vi "SPS Flow System Automation.vi"() -> ()   [LabVIEW 2018]
uses:
  Serial configuration cluster control.ctl
  SPS Flow System Automation Control.ctl
  <vilib>/Utility/miscctls.llb/LVRowAndColumnTypeDef.ctl
panel:
  out "Path to ConditionTable (*.txt)":path caption="selected path"
  in  "Left Syringe Type":u16(ring)=2500 items=["Yellow Syringes"=50, "Green Syringes"=250, "Blue Syringes"=500, "Red Syringes"=2500]
  in  "Right Syringe Type":u16(ring)=500 items=["Yellow Syringes"=50, "Green Syringes"=250, "Blue Syringes"=500, "Red Syringes"=2500]
  out "State":T1=enum."Check temp & time "
  in  "Simulate Right Pump":i32(ring)=2 items=["Error"=-1, "Unitialised"=0, "Initialising"=1, "Idle"=2, "Filling"=3, "Full"=4, "Emptying"=5, "Empty"=6, "Pumping"=7]
  out "Pump2-2":bool
  out "Status":i32(ring) items=["Error"=-1, "Unitialised"=0, "Initialising"=1, "Idle"=2, "Filling"=3, "Full"=4, "Emptying"=5, "Empty"=6, "Pumping"=7]
  out "Pump2-1":bool
  in  "Waste Port (Valve 4)":u32=1
  out "Flow Rate\n(ml/min)":sgl
  in  "Temp range":dbl=5.0 caption="Temp(°C) Range ±"
  out "Asia pump connection":i32
  in  "Simulate Left Pump":i32(ring)=2 items=["Error"=-1, "Unitialised"=0, "Initialising"=1, "Idle"=2, "Filling"=3, "Full"=4, "Emptying"=5, "Empty"=6, "Pumping"=7]
  out "Flow Rate\n(ml/min)":sgl
  out "Status":i32(ring) items=["Error"=-1, "Unitialised"=0, "Initialising"=1, "Idle"=2, "Filling"=3, "Full"=4, "Emptying"=5, "Empty"=6, "Pumping"=7]
  out "Valve 4":u32(knob) scale=10.0..1.0
  out "Current Temp":dbl(slide) scale=10.0..150.0
  out "Pump1":bool
  in  "Valve pos reached":bool
  in  "temp reached":bool
  in  "Starting from row":i32=1
  out "Conditions Table":string[][](table)=[["1-1 1st reaction", "0.5", "2", "2", "0", "0", "10", "1", "1", "off", "off"], ["1-2 heating", "x", "0", "2", "0", "0", "10", "1", "1", "32", "500"], ["1-2 1st reaction", "0.5", "4", "2", "0", "0", "10", "1", "1", "32", "500"], ["1-3 DCM wash", "0.5", "5", "1", "0", "0", "10", "2", "1", "off", "off"], ["1-4 MeOH wash", "0.5", "2", "7", "0", "0", "10", "2", "1", "off", "off"], ["1-5 N2 purge", "0.5", "0", "6", "0", "0", "10", "2", "10", "off", "off"], ["1-6 THF wash", "0.5", "1", "6", "1", "1", "10", "2", "1", "off", "off"], ["1-7 THF wash", "0.5", "2", "6", "3", "1", "10", "2", "1", "off", "off"], ["2-1 2nd mixing", "0.5", "2.5", "3", "2.5", "0", "9", "3", "1", "off", "off"], ["2-2 heating", "x", "0", "4", "0", "0", "9", "3", "1", "38", "500"], ["2-3 2nd reaction", "0.5", "3", "4", "0", "0", "9", "3", "1", "38", "500"], ["2-5 THF wash", "0.5", "2", "6", "1", "1", "10", "2", "1", "38", "500"], ["2-4 N2 purge", "0.5", "0", "6", "0", "0", "10", "2", "10", "38", "500"], ["2-6 cooling", "x", "0", "6", "0", "0", "10", "2", "1", "30", "500"], ["2-7 THF wash", "0.5", "2.5", "6", "2.5", "1", "10", "2", "1", "off", "off"], ["3-1 3rd reaction", "0.5", "2.5", "5", "0", "2.5", "1", "2", "1", "off", "off"], ["3-3 THF wash", "0.5", "2.5", "6", "1", "2.5", "10", "2", "1", "off", "off"], ["3-4 0.5 N HCl wash", "0.5", "0", "6", "5", "0", "7", "2", "1", "off", "off"], ["3-6 heating", "x", "0", "6", "0", "0", "7", "2", "1", "60", "500"], ["3-7 H2O wash", "20", "0", "6", "5", "0", "8", "2", "1", "60", "500"], ["3-8 THF wash", "15", "0", "6", "4", "1", "10", "2", "1", "60", "500"], ["4-1 EtOH-THF wash", "20", "0", "6", "2.5", "0", "3", "2", "1", "60", "500"], ["4-1 heating", "x", "0", "6", "0", "0", "3", "5", "1", "110", "500"], ["4-3 4th reaction", "360", "0", "6", "2.5", "0", "2", "4", "1", "110", "500"], ["4-4 EtOH-THF wash ", "20", "0", "6", "2.5", "0", "3", "5", "1", "110", "500"], ["4-5 THF wash  ", "20", "1.5", "6", "2.5", "1", "10", "5", "1", "110", "500"], ["4-6 N2 purge", "20", "0", "6", "0", "0", "10", "2", "10", "110", "500"], ["5-1 Dioxane-DMSO wash", "20", "2.5", "15", "2.5", "0", "4", "5", "1", "110", "500"], ["5-2 5th mixing", "12", "2.5", "14", "2.5", "0", "5", "6", "1", "110", "500"], ["5-3 5th reaction", "600", "0", "14", "2.5", "0", "6", "6", "1", "110", "500"], ["5-4 MeOH & THF wash", "20", "2.5", "7", "1.5", "1", "10", "5", "1", "off", "off"], ["5-5 N2 purge", "20", "0", "7", "0", "0", "10", "2", "10", "off", "off"], ["6-1 DCM wash", "15", "2", "1", "0", "0", "10", "2", "1", "off", "off"], ["6-2 DCM wash", "20", "5", "1", "0", "0", "10", "2", "1", "off", "off"], ["6-4 6th reaction", "60", "3", "16", "0", "0", "10", "7", "1", "off", "off"], ["6-5 DCM wash", "10", "5", "1", "0", "0", "10", "7", "1", "off", "off"], ["", "", "", "", "", "", "", "", "", "", ""], ["", "", "", "", "", "", "", "", "", "", ""], ["", "", "", "", "", "", "", "", "", "", ""], ["", "", "", "", "", "", "", "", "", "", ""], ["", "", "", "", "", "", "", "", "", "", ""], ["", "", "", "", "", "", "", "", "", "", ""], ["", "", "", "", "", "", "", "", "", "", ""], ["", "", "", "", "", "", "", "", "", "", ""], ["", "", "", "", "", "", "", "", "", "", ""], ["", "", "", "", "", "", "", "", "", "", ""], ["", "", "", "", "", "", "", "", "", "", ""], ["", "", "", "", "", "", "", "", "", "", ""], ["", "", "", "", "", "", "", "", "", "", ""], ["", "", "", "", "", "", "", "", "", " ", ""]]
  in  "Pause":bool
  out "Valve 3":u32(knob) scale=16.0..1.0
  out "Valve 2":u32(knob) scale=10.0..1.0
  out "Valve 1":u32(knob) scale=16.0..1.0
  out "Total numer of rows":i32=50
  out "Row No.":i32=1
  in  "Serial Configuration":T2(tab)=enum."Stir Plate"
  in  "Valve 1 Serial Config":T3={"Baud Rate"=9600, "Parity"=0, "Data Bits"=8, "VISA resource name"=""} {"Data Bits" items=["7"=7, "8"=8]; "Parity" items=["None", "Odd", "Even"]; "Baud Rate" items=["300"=300, "600"=600, "1200"=1200, "2400"=2400, "4800"=4800, "9600"=9600, "19200"=19200]}
  in  "Valve 2 Serial Config":T3={"Baud Rate"=9600, "Parity"=0, "Data Bits"=8, "VISA resource name"=""} {"Data Bits" items=["7"=7, "8"=8]; "Parity" items=["None", "Odd", "Even"]; "Baud Rate" items=["300"=300, "600"=600, "1200"=1200, "2400"=2400, "4800"=4800, "9600"=9600, "19200"=19200]}
  in  "Valve 3 Serial Config":T3={"Baud Rate"=9600, "Parity"=0, "Data Bits"=8, "VISA resource name"=""} {"Data Bits" items=["7"=7, "8"=8]; "Parity" items=["None", "Odd", "Even"]; "Baud Rate" items=["300"=300, "600"=600, "1200"=1200, "2400"=2400, "4800"=4800, "9600"=9600, "19200"=19200]}
  in  "Valve 4 Serial Config":T3={"Baud Rate"=9600, "Parity"=0, "Data Bits"=8, "VISA resource name"=""} {"Data Bits" items=["7"=7, "8"=8]; "Parity" items=["None", "Odd", "Even"]; "Baud Rate" items=["300"=300, "600"=600, "1200"=1200, "2400"=2400, "4800"=4800, "9600"=9600, "19200"=19200]}
  in  "Pump 1 Serial Config":T3={"Baud Rate"=9600, "Parity"=0, "Data Bits"=8, "VISA resource name"=""} {"Data Bits" items=["7"=7, "8"=8]; "Parity" items=["None", "Odd", "Even"]; "Baud Rate" items=["300"=300, "600"=600, "1200"=1200, "2400"=2400, "4800"=4800, "9600"=9600, "19200"=19200]}
  in  "Hotplate Serial Config":T3={"Baud Rate"=9600, "Parity"=2, "Data Bits"=7, "VISA resource name"=""} {"Data Bits" items=["7"=7, "8"=8]; "Parity" items=["None", "Odd", "Even"]; "Baud Rate" items=["300"=300, "600"=600, "1200"=1200, "2400"=2400, "4800"=4800, "9600"=9600, "19200"=19200]}
  out "Elapsed Time":dbl=0.21800044377644856 caption="Elapsed Time (s)" format="%#.2g"
  in  "Start":bool
  in  "stop":bool
  # "Debugging"
  # "Parameters Setup"
  # "Condition Table"
  # "Current Status"
  # "!!! Avoid aborting the program when Pump2 is initializing !!!"
  # "(min)"
  # "°C"
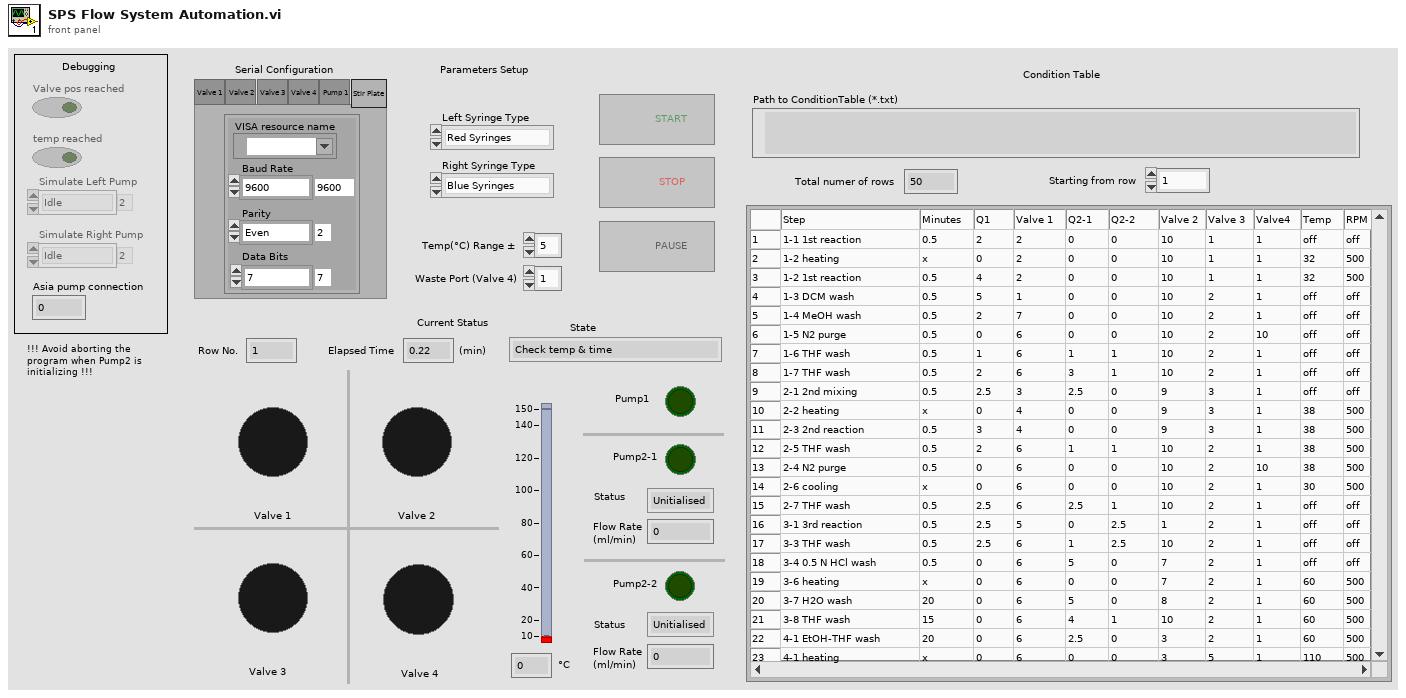
[diagram p1: front panel]
types:
  T1 = typedef "SPS Flow System Automation Control.ctl" = enum16{"Start operation", "Initialize", "Wait to start", "Set valves position", "Turn on heating", "Wait to reach temp", "Fill syringe pump", "Start pumps", "Check temp & time ", "Pause pumps ", "Resume pumps", "Stop pumps", "Empty syringe pump", "Check next step", "No more entries"}
  T2 = enum32{"Valve 1", "Valve 2", "Valve 3", "Valve 4", "Pump 1", "Stir Plate"}
  T3 = typedef "Serial configuration cluster control.ctl" = cluster{"Baud Rate":u32, "Parity":u16, "Data Bits":u16, "VISA resource name":refnum<visa-resource-name>}
  T4 = enum8{"Enabled", "Disabled", "Disabled and Grayed Out"}
  T5 = typedef "LVRowAndColumnTypeDef.ctl" = cluster{"Row":i32, "Column":i32}
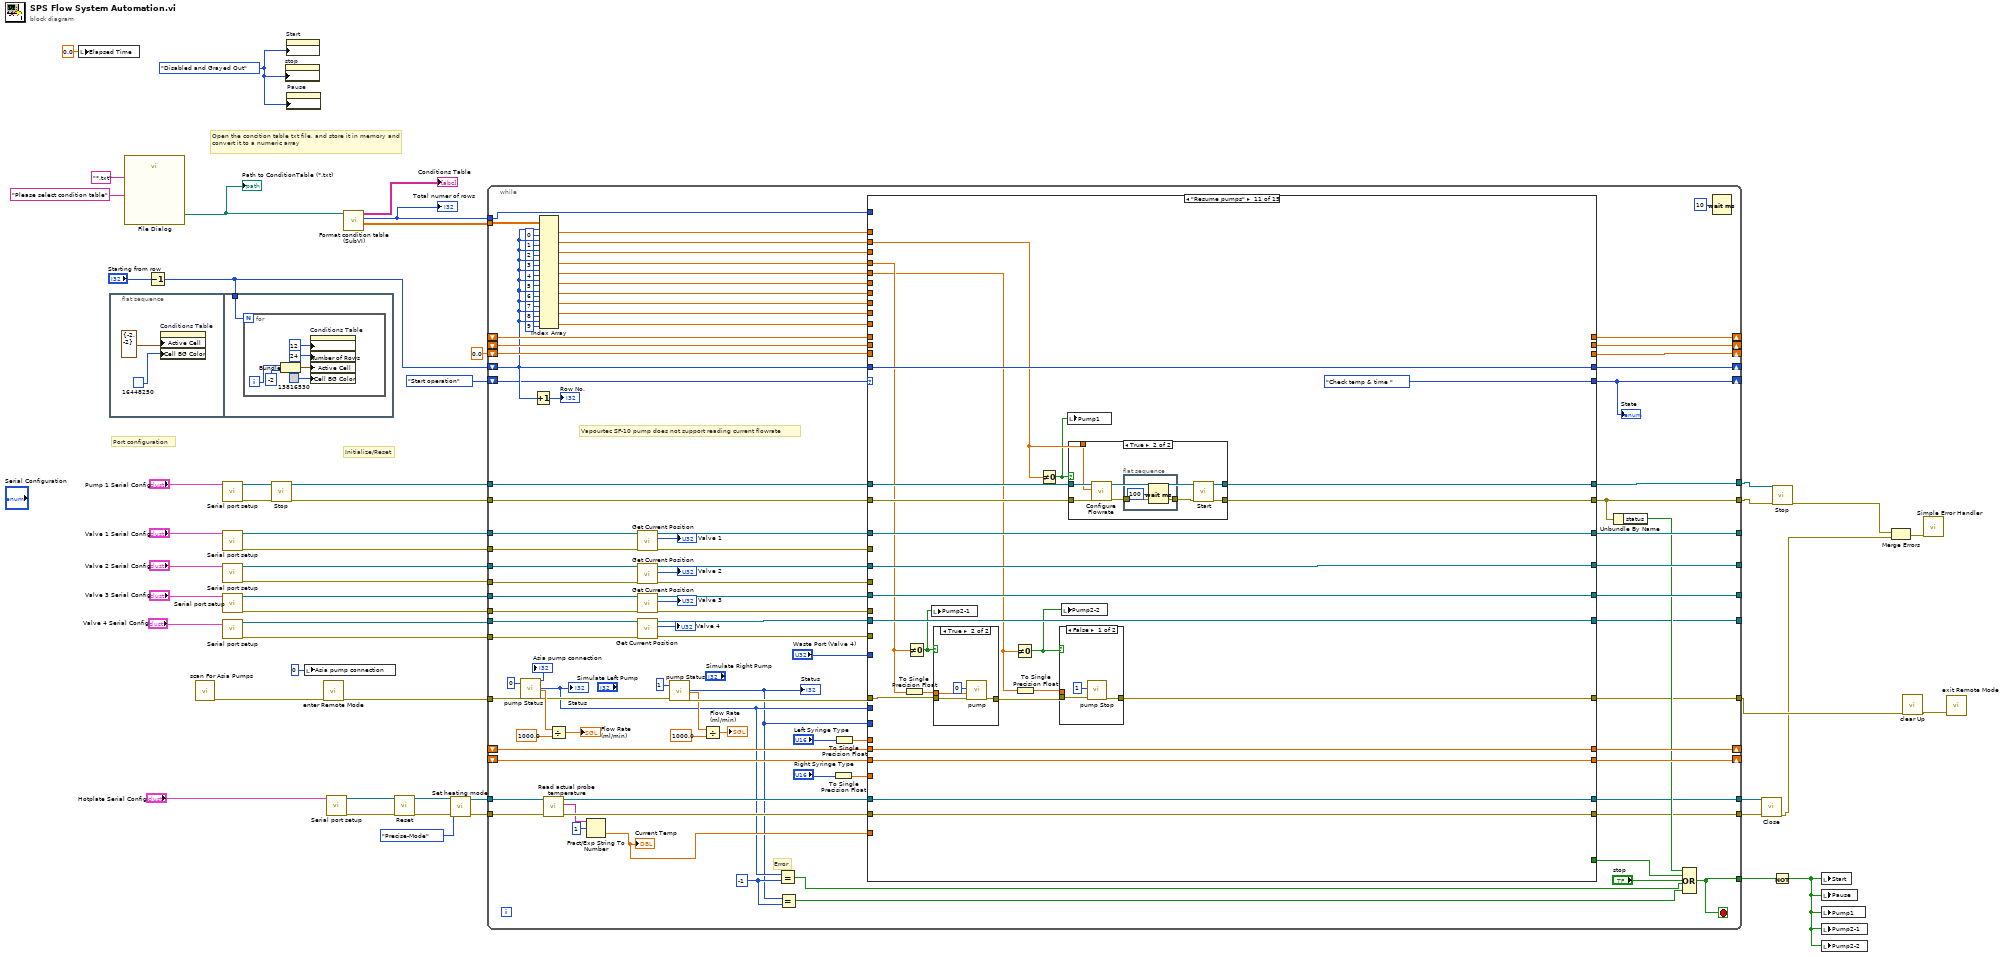
[diagram p0: block diagram]
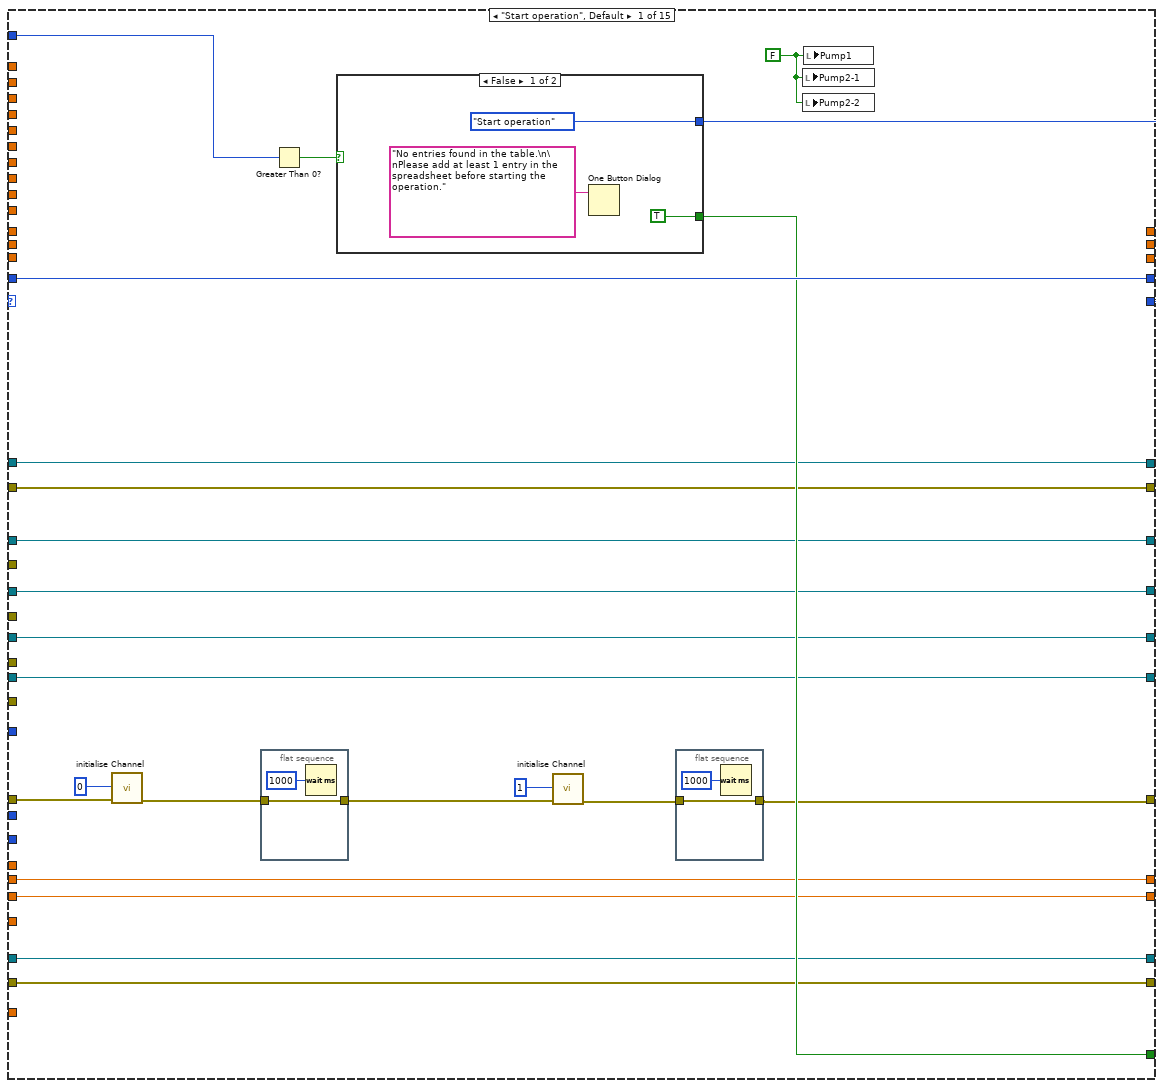
[diagram p2: hidden frame]
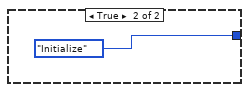
[diagram p3: hidden frame]
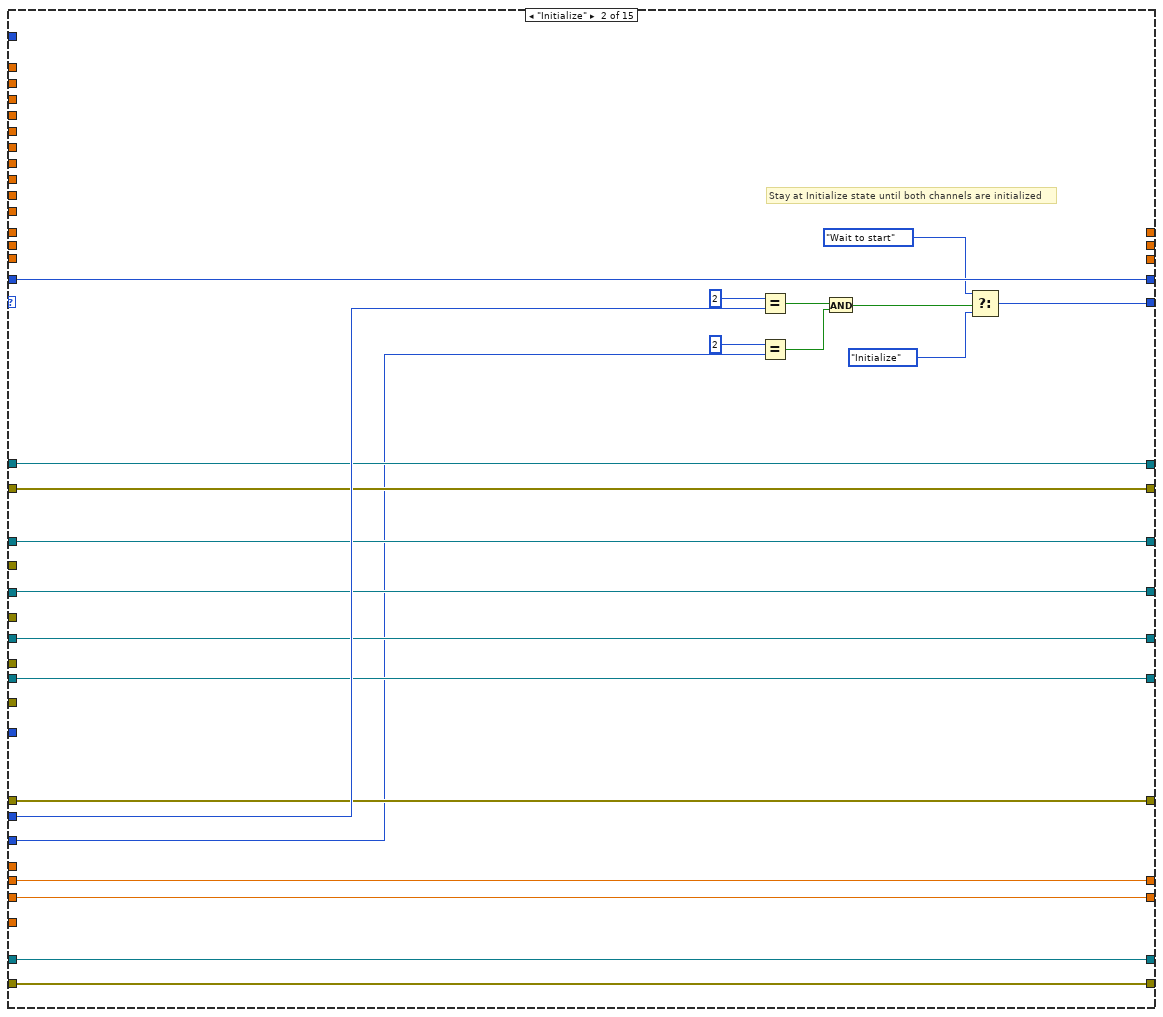
[diagram p4: hidden frame]
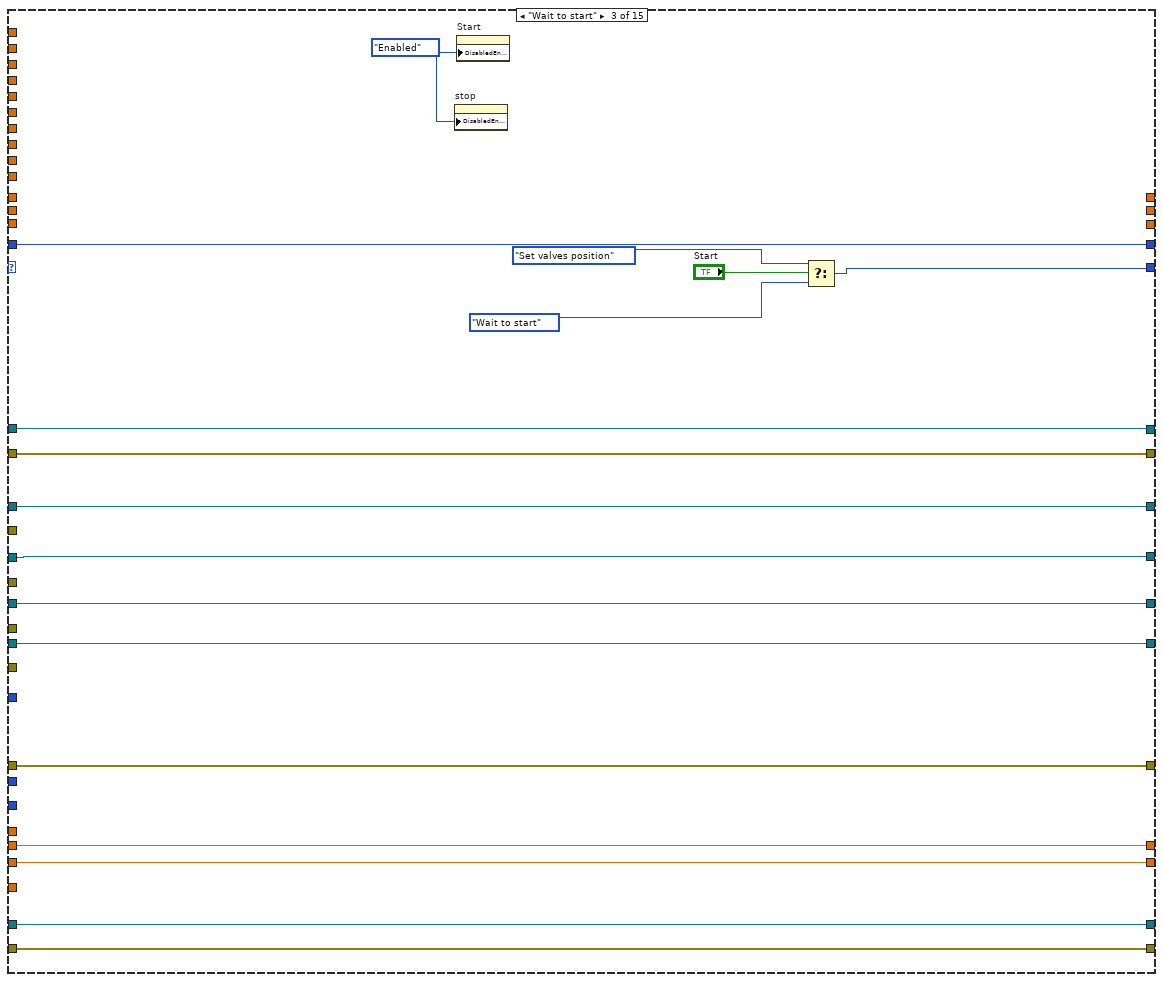
[diagram p5: hidden frame]
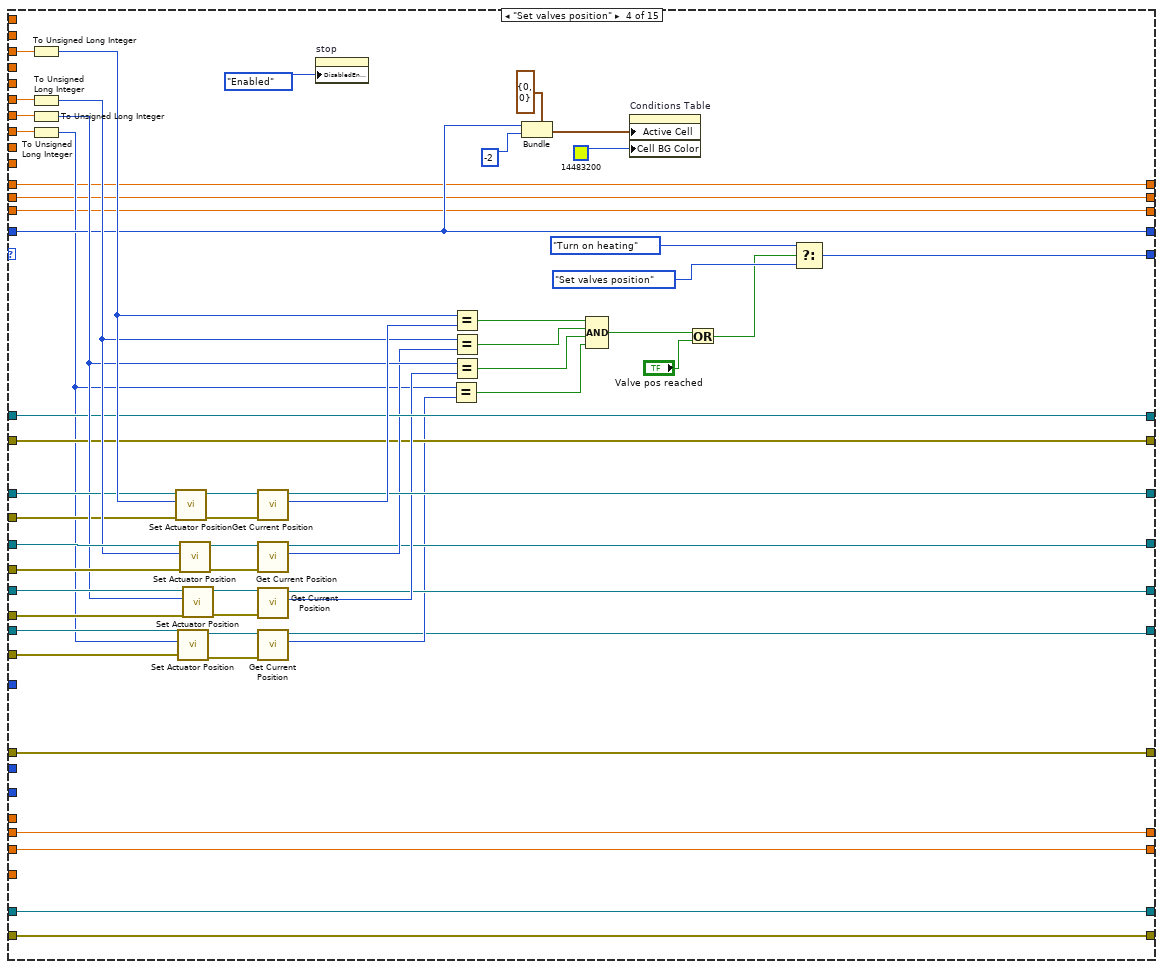
[diagram p6: hidden frame]
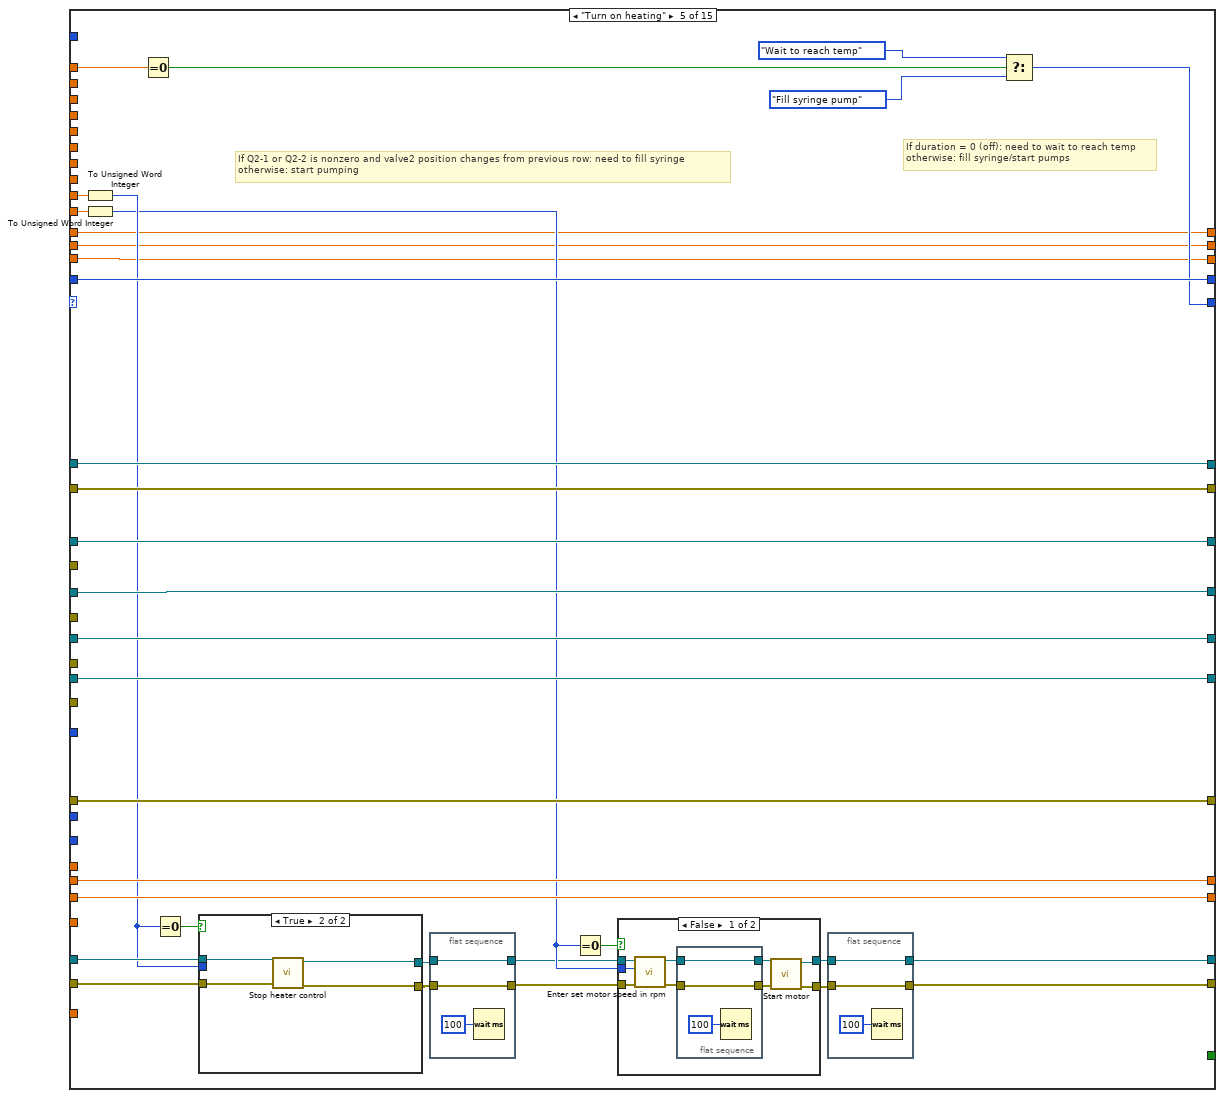
[diagram p7: hidden frame]
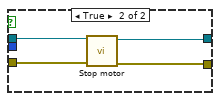
[diagram p8: hidden frame]
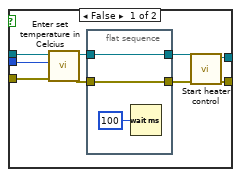
[diagram p9: hidden frame]
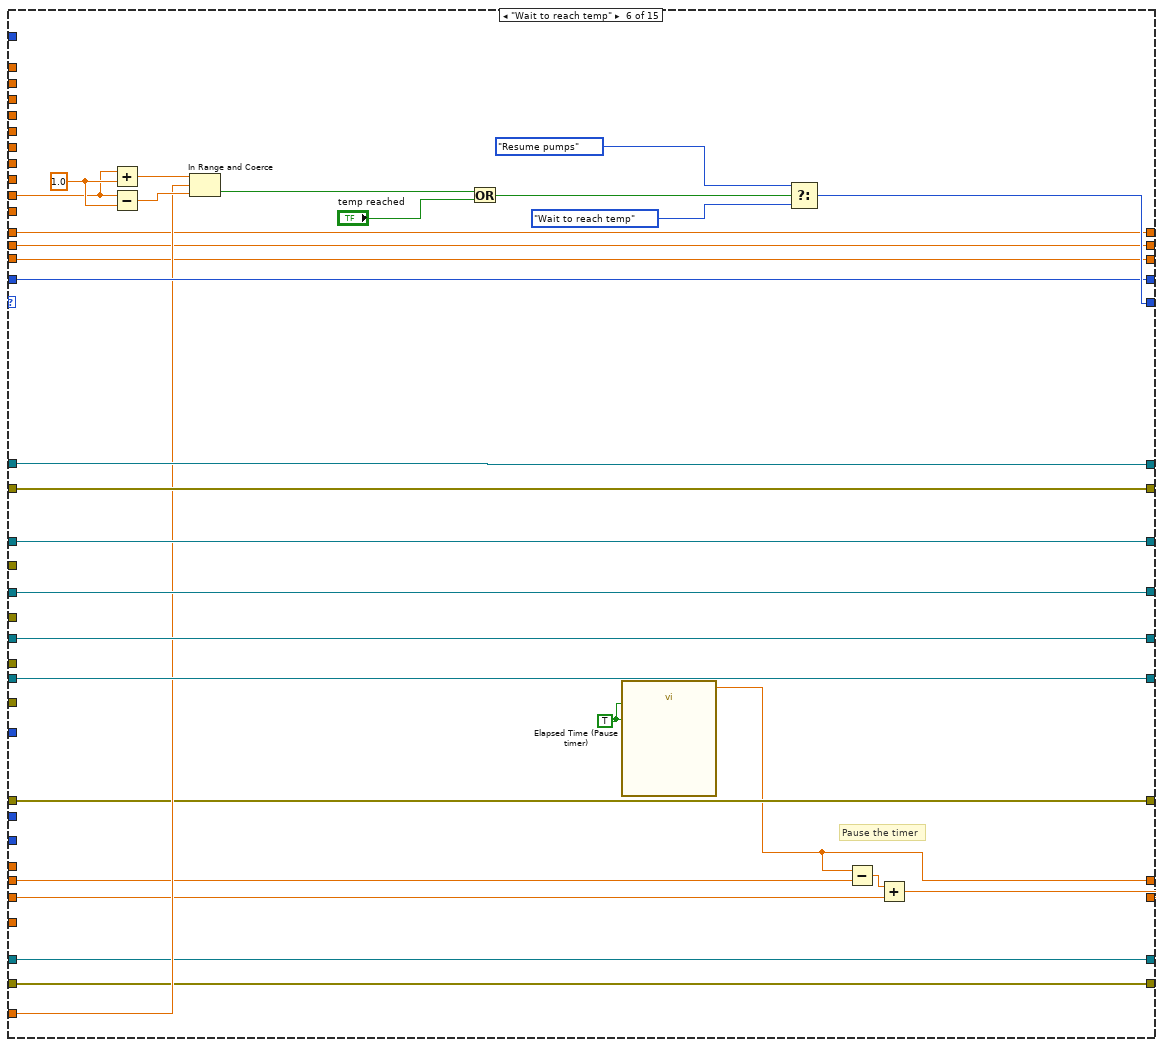
[diagram p10: hidden frame]
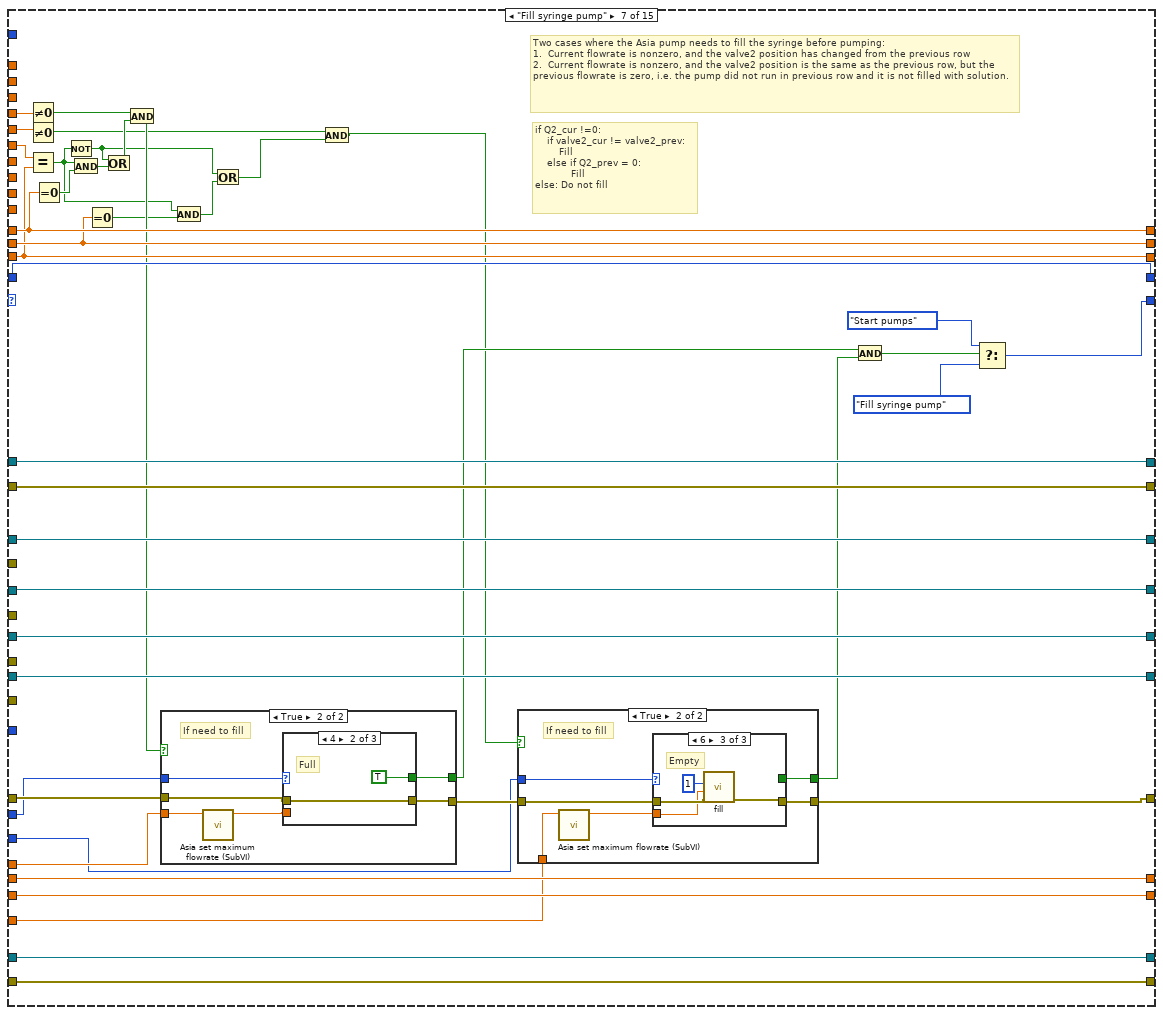
[diagram p11: hidden frame]
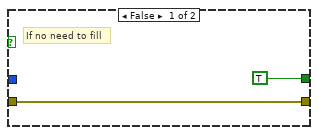
[diagram p12: hidden frame]
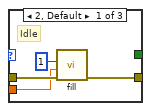
[diagram p13: hidden frame]
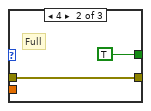
[diagram p14: hidden frame]
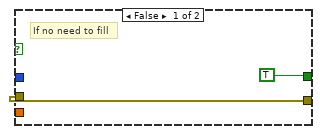
[diagram p15: hidden frame]
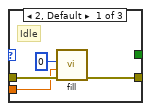
[diagram p16: hidden frame]
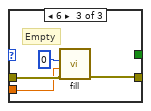
[diagram p17: hidden frame]
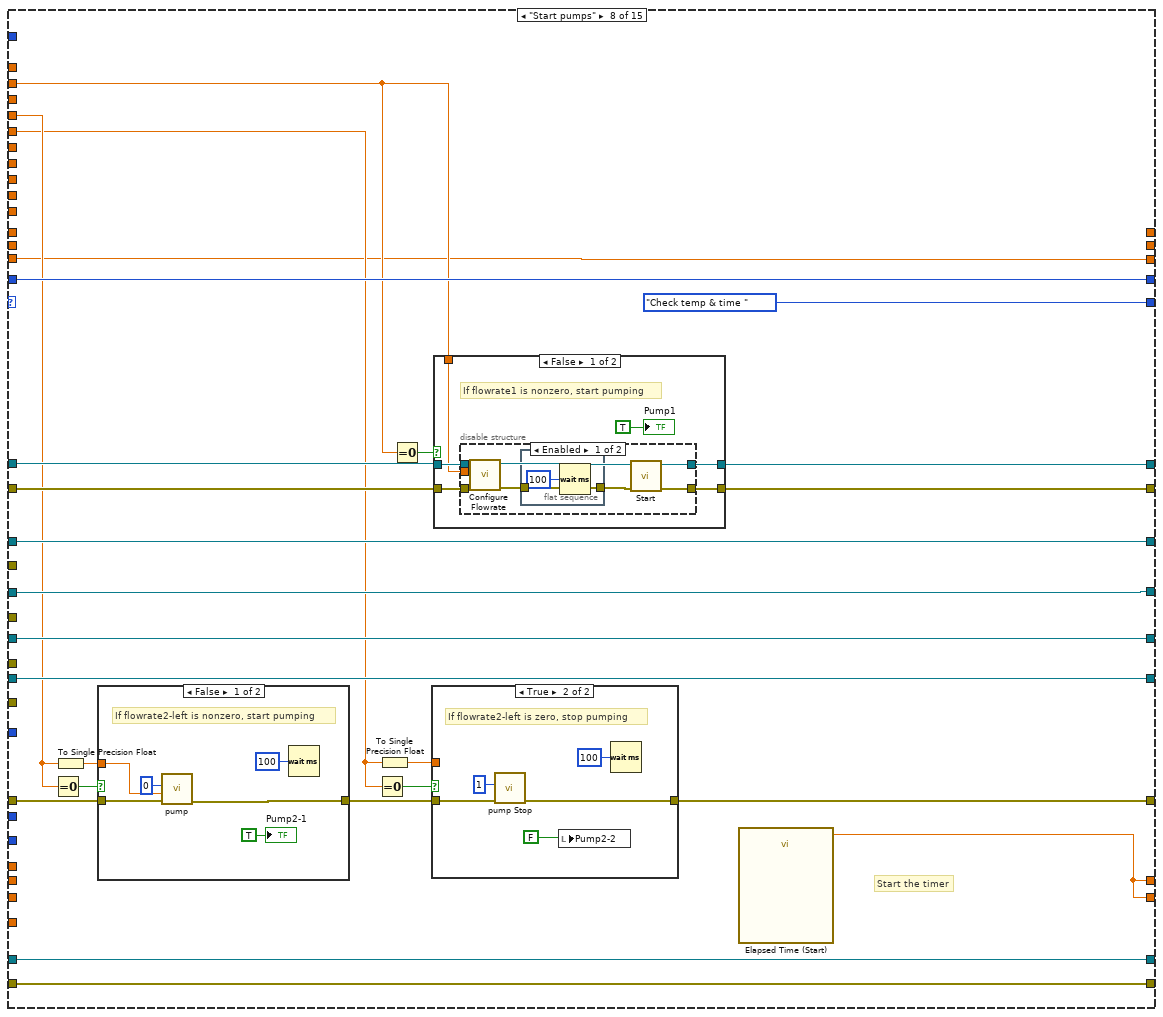
[diagram p18: hidden frame]
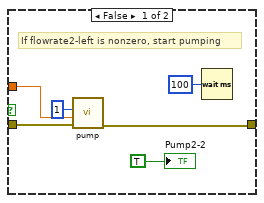
[diagram p19: hidden frame]
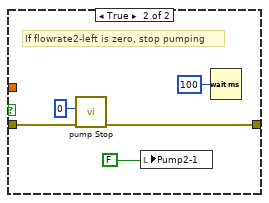
[diagram p20: hidden frame]
diagram:
  w22 = T4."Disabled and Grayed Out" ("Disabled")
  # "Open the concition table txt file, and store it in memory and convert it to a numeric array"
  # "Initialize/Reset"
  # "Port configuration"
  n1 = local write "Elapsed Time"(0.0 ("Elapsed Time")) -> ()
  n2 = flat-sequence {
    tunnel: w33 -> [w54]
    frame #0 {
      n3 = property on="Conditions Table" class="Tbl (strict)"("Active Cell"=T5 {"Row"=-2, "Column"=-2} ("Active Cell:Active Cell"), "Cell BG Color"=u32 16448250) -> ()  [unwired: 2 in, 2 out]
    }
    frame #1 {
      n4 = for {
        N: w54 -> [_]
        i -> [w56]
        n5 = Bundle(w56, "index"=-2) -> (w55:cluster{i32, "index":i32})  [unwired: 1 in]
        n6 = property on="Conditions Table" class="Tbl (strict)"("Number of Columns"=u32 12, "Number of Rows"=u32 24 ("Number of Columns"), "Active Cell"=w55, "Cell BG Color"=u32 13816530) -> ()  [unwired: 2 in, 2 out]
      }
    }
  }
  n7 = call "File Dialog"("prompt"="Please select condition table", "pattern (all files)"="*.txt") -> ("selected path"=w14:path)  [unwired: 10 in, 3 out]
  "Path to ConditionTable (*.txt)" <- w14
  n8 = Decrement(x="Starting from row") -> (x-1=w33:i32)
  n9 = call "scan For Asia Pumps.vi"() -> ("error out"=w26:errorcluster)  [unwired: 10 in, 1 out]
  n10 = call "Serial port setup.vi"("Serial Configuration"="Pump 1 Serial Config") -> ("error out"=w9:errorcluster, "VISA resource name out"=w10:refnum<visa-resource-name>)  [unwired: 9 in]
  n11 = call "Serial port setup.vi"("Serial Configuration"="Valve 1 Serial Config") -> ("error out"=w44:errorcluster, "VISA resource name out"=w47:refnum<visa-resource-name>)  [unwired: 9 in]
  n12 = call "Serial port setup.vi"("Serial Configuration"="Valve 2 Serial Config") -> ("error out"=w24:errorcluster, "VISA resource name out"=w25:refnum<visa-resource-name>)  [unwired: 9 in]
  n13 = call "Serial port setup.vi"("Serial Configuration"="Valve 3 Serial Config") -> ("error out"=w45:errorcluster, "VISA resource name out"=w46:refnum<visa-resource-name>)  [unwired: 9 in]
  n14 = call "Serial port setup.vi"("Serial Configuration"="Valve 4 Serial Config") -> ("error out"=w30:errorcluster, "VISA resource name out"=w31:refnum<visa-resource-name>)  [unwired: 9 in]
  n15 = call "Stop.vi"("error in (no error)"=w9, "VISA resource name"=w10) -> ("error out"=w41:errorcluster, "VISA resource name out"=w42:refnum<visa-resource-name>)  [unwired: 8 in]
  n16 = property on="stop" class="Bool"("DisabledEnum"=w22) -> ()  [unwired: 2 in, 2 out]
  n17 = property on="Start" class="Bool (strict)"("DisabledEnum"=w22) -> ()  [unwired: 2 in, 2 out]
  n18 = property on="Pause" class="Bool (strict)"("DisabledEnum"=w22) -> ()  [unwired: 2 in, 2 out]
  n19 = local write "Asia pump connection"(0 ("Asia pump connection")) -> ()
  n20 = call "enter Remote Mode.vi"("error in (no error)"=w26) -> ("error out"=w17:errorcluster)  [unwired: 9 in, 1 out]
  n21 = call "Serial port setup.vi"("Serial Configuration"="Hotplate Serial Config") -> ("error out"=w7:errorcluster, "VISA resource name out"=w8:refnum<visa-resource-name>)  [unwired: 9 in]
  n22 = call "Format condition table (SubVI).vi"("file path (use dialog)"=w14) -> ("Reformated table"=w21:dbl[][], "Number of rows"=w43:i32, "Conditions Table"=→"Conditions Table":string[][])  [unwired: 8 in]
  "Total numer of rows" <- w43
  n23 = call "Reset.vi"("error in (no error)"=w7, "VISA resource name"=w8) -> ("error out"=w5:errorcluster, "VISA resource name out"=w6:refnum<visa-resource-name>)  [unwired: 8 in]
  n24 = call "Set heating mode.vi"("error in (no error)"=w5, "MODE"=enum16{"Precise-Mode", "Fast-Mode"}."Precise-Mode", "VISA resource name"=w6) -> ("error out"=w28:errorcluster, "VISA resource name out"=w29:refnum<visa-resource-name>)  [unwired: 7 in]
  n25 = while {
    tunnel: w21 -> [w156]
    tunnel: w47 -> [w141]
    tunnel: w25 -> [w139]
    tunnel: w46 -> [w137]
    tunnel: w45 -> [w129]
    tunnel: w24 -> [w131]
    tunnel: w44 -> [w133]
    shift-right: [w152] -> _
    shift-left: w33 -> [w69]
    tunnel: w42 -> [w70]
    tunnel: w41 -> [w148]
    tunnel: w43 -> [w144]
    tunnel: [w143] -> _
    tunnel: [w142] -> w40
    tunnel: [w135] -> _
    tunnel: [w134] -> _
    tunnel: [w126] -> w39
    tunnel: [w127] -> w38
    shift-right: [w125] -> _
    shift-left: _ -> [w109]
    shift-right: [w124] -> _
    shift-left: _ -> [w108]
    tunnel: w31 -> [w121]
    tunnel: w30 -> [w120]
    tunnel: [w117] -> _
    tunnel: w29 -> [w113]
    tunnel: w28 -> [w112]
    tunnel: [w105] -> w1
    tunnel: [w104] -> w2
    tunnel: w17 -> [w103]
    shift-right: [w102] -> _
    shift-left: 0.0 ("String") -> [w101]
    tunnel: [w100] -> w19
    shift-right: [w76] -> _
    shift-left: _ -> [w75]
    shift-right: [w77] -> _
    shift-left: _ -> [w74]
    shift-right: [w67] -> _
    shift-left: SPS_Flow_System_Automation_Control."Start operation" -> [w68]
    stop <- w127 stop-if-true
    w79 = -1 ("y")
    # "Error"
    # "Vapourtec SF-10 pump does not support reading current flowrate"
    n26 = call "pump Status.vi"("channel"=u32 0, "error in (no error)"=w103) -> ("function return"=→"Asia pump connection":i32, "pumpState out"=w73:i32, "pumpRate out"=w98:sgl, "error out"=w92:errorcluster)  [unwired: 19 in, 3 out]
    "Status" <- w73
    n27 = Increment(x=w69) -> (x+1=→"Row No.":i32)
    n28 = Index Array(array=w156, index (row) #1=w69, index (col) #1=0 ("disabled index (col)"), index (row) #2=w69, index (col) #2=1 ("disabled index (col)"), index (row) #3=w69, index (col) #3=2 ("disabled index (col)"), index (row) #4=w69, index (col) #4=3 ("disabled index (col)"), index (row) #5=w69, index (col) #5=4 ("disabled index (col)"), index (row) #6=w69, index (col) #6=5 ("disabled index (col)"), index (row) #7=w69, index (col) #7=6 ("index (col)"), index (row) #8=w69, index (col) #8=7 ("index (col)"), index (row) #9=w69, index (col) #9=8 ("disabled index (col)"), index (row) #10=w69, index (col) #10=9 ("index (col)")) -> (element #1=w146:dbl, element #2=w147:dbl, element #3=w151:dbl, element #4=w145:dbl, element #5=w150:dbl, element #6=w149:dbl, element #7=w114:dbl, element #8=w115:dbl, element #9=w106:dbl, element #10=w81:dbl)
    n29 = call "Read actual probe temperature.vi"("error in (no error)"=w112, "VISA resource name"=w113) -> ("error out"=w110:errorcluster, "read buffer"=w65:string, "VISA resource name out"=w111:refnum<visa-resource-name>)  [unwired: 7 in]
    n30 = Divide(x=w98, y=sgl 1000.0) -> (x/y=→"Flow Rate\n(ml/min)":sgl)
    n31 = Fract/Exp String To Number(string=w65, offset=1) -> (number=w78:dbl)  [unwired: 2 in, 1 out]
    "Current Temp" <- w78
    n32 = call "Get Current Position.vi"("error in (no error)"=w133, "VISA resource name"=w141) -> ("error out"=w132:errorcluster, "Current Position out"=→"Valve 1":u32, "VISA resource name out"=w140:refnum<visa-resource-name>)  [unwired: 7 in]
    n33 = call "Get Current Position.vi"("error in (no error)"=w131, "VISA resource name"=w139) -> ("error out"=w130:errorcluster, "Current Position out"=→"Valve 2":u32, "VISA resource name out"=w138:refnum<visa-resource-name>)  [unwired: 7 in]
    n34 = call "Get Current Position.vi"("error in (no error)"=w129, "VISA resource name"=w137) -> ("error out"=w128:errorcluster, "Current Position out"=→"Valve 3":u32, "VISA resource name out"=w136:refnum<visa-resource-name>)  [unwired: 7 in]
    n35 = call "Get Current Position.vi"("error in (no error)"=w120, "VISA resource name"=w121) -> ("error out"=w119:errorcluster, "Current Position out"=→"Valve 4":u32, "VISA resource name out"=w118:refnum<visa-resource-name>)  [unwired: 7 in]
    n36 = call "pump Status.vi"("channel"=u32 1, "error in (no error)"=w92) -> ("pumpState out"=w72:i32, "pumpRate out"=w87:sgl, "error out"=w91:errorcluster)  [unwired: 19 in, 4 out]
    "Status" <- w72
    n37 = Divide(x=w87, y=sgl 1000.0) -> (x/y=→"Flow Rate\n(ml/min)":sgl)
    n38 = Equal?(x=w73, y=w79) -> (x = y?=w99:bool)
    n39 = Equal?(x=w72, y=w79) -> (x = y?=w85:bool)
    n40 = To Single Precision Float(number="Right Syringe Type") -> (single precision float=w83:sgl)
    n41 = To Single Precision Float(number="Left Syringe Type") -> (single precision float=w93:sgl)
    n42 = case shown="\"Resume pumps\"" w68 {
      tunnel: [w183 w213 w216 w247 w306 w392 w411 SPS_Flow_System_Automation_Control."Check temp & time " w567 w611 SPS_Flow_System_Automation_Control."Check temp & time " SPS_Flow_System_Automation_Control."Empty syringe pump" w747 w890 SPS_Flow_System_Automation_Control."No more entries"] -> w67
      tunnel: [w181 _ _ _ _ _ _ _ _ _ _ _ _ _ TRUE] -> w154
      tunnel: w140 -> [w180 w209 w231 w281 w323 w389 w431 w492 w583 w622 w670 w727 w771 w886 w912]
      tunnel: w138 -> [w178 w208 w229 w289 w321 w387 w430 w491 w581 w620 w669 w726 w764 w885 w911]
      tunnel: w136 -> [w177 w206 w228 w288 w320 w386 w429 w490 w580 w619 w668 w725 w770 w884 w910]
      tunnel: w128 -> [_ _ _ w287 _ _ _ _ _ _ _ _ _ _ _]
      tunnel: w130 -> [_ _ _ w286 _ _ _ _ _ _ _ _ _ _ _]
      tunnel: w69 -> [w182 w212 w232 w265 w324 w390 w434 w495 w587 w617 w671 w722 w774 w889 w916]
      tunnel: [w182 w212 w232 w265 w324 w390 w434 w495 w587 w617 w671 w720 w774 w889 w916] -> w152
      tunnel: w151 -> [_ _ _ w284 _ _ _ _ _ _ _ _ _ _ _]
      tunnel: w150 -> [_ _ _ _ _ _ w409 w474 _ _ w655 w700 w742 w876 _]
      tunnel: w149 -> [_ _ _ w244 _ _ w406 _ _ _ _ w708 w763 _ _]
      tunnel: w115 -> [_ _ _ w246 _ _ _ _ _ _ _ _ _ _ _]
      tunnel: w70 -> [w179 w211 w230 w277 w322 w388 w433 w494 w582 w624 w666 w719 w773 w888 w914]
      tunnel: w148 -> [w176 w210 w227 w270 w319 w385 w432 w493 w579 w623 w665 w717 w772 w887 w913]
      tunnel: w147 -> [_ _ _ _ _ _ _ w485 _ _ w662 _ _ w896 _]
      tunnel: w146 -> [_ _ _ _ w309 _ _ _ w585 _ _ _ _ w897 _]
      tunnel: w145 -> [_ _ _ _ _ _ w410 w478 _ _ w656 w701 w741 w895 _]
      tunnel: w144 -> [w185 _ _ _ _ _ _ _ _ _ _ _ _ _ _]
      tunnel: [w180 w209 w231 w279 w323 w389 w431 w492 w583 w622 w670 w727 w771 w886 w912] -> w143
      tunnel: [w179 w211 w230 w277 w322 w388 w433 w484 w582 w621 w663 w718 w773 w888 w914] -> w142
      tunnel: [w178 w208 w229 w272 w321 w387 w430 w491 w581 w620 w669 w726 w764 w885 w911] -> w135
      tunnel: [w177 w206 w228 w271 w320 w386 w429 w490 w580 w619 w668 w725 w770 w884 w910] -> w134
      tunnel: [w176 w210 w227 w270 w319 w385 w432 w483 w579 w618 w664 w716 w772 w887 w913] -> w126
      tunnel: w132 -> [_ _ _ w264 _ _ _ _ _ _ _ _ _ _ _]
      tunnel: [w174 w204 w225 w253 w317 w372 w427 w489 w577 w604 w660 w714 w769 w881 w907] -> w125
      tunnel: [w173 w203 w224 w252 w316 w369 w426 w489 w576 w602 w659 w713 w768 w880 w906] -> w124
      tunnel: w119 -> [_ _ _ w258 _ _ _ _ _ _ _ _ w761 _ _]
      tunnel: w118 -> [w175 w207 w226 w259 w318 w379 w428 w488 w566 w616 w661 w715 w762 w883 w909]
      tunnel: [w175 w207 w226 w254 w318 w379 w428 w488 w566 w616 w661 w715 w755 w883 w909] -> w117
      tunnel: w114 -> [_ _ _ w245 _ _ _ _ _ _ _ _ _ _ _]
      tunnel: w111 -> [w172 w202 w223 w251 w315 w377 w425 w487 w565 w615 w658 w711 w767 w879 w905]
      tunnel: w110 -> [w171 w201 w222 w250 w314 w376 w424 w486 w564 w614 w657 w712 w766 w878 w904]
      tunnel: w109 -> [w174 w204 w225 w253 w317 w371 w427 _ w561 w605 w660 w714 w769 w881 w907]
      tunnel: w108 -> [w173 w203 w224 w252 w316 w370 w426 _ w563 w603 w659 w713 w768 w880 w906]
      tunnel: [w172 w202 w223 w251 w313 w377 w425 w487 w565 w615 w658 w711 w767 w879 w905] -> w105
      tunnel: [w171 w201 w222 w250 w312 w376 w424 w486 w564 w614 w657 w712 w766 w878 w904] -> w104
      tunnel: w106 -> [_ _ _ _ w303 w366 _ _ w557 _ _ _ _ w877 _]
      tunnel: w78 -> [_ _ _ _ _ w378 _ _ w562 _ _ _ _ _ _]
      tunnel: w91 -> [w170 w205 w221 w248 w311 w374 w422 w477 w560 w613 w653 w710 w745 w882 w903]
      tunnel: w73 -> [_ w215 _ _ _ _ w418 _ _ _ _ _ w756 _ _]
      tunnel: [_ _ _ w243 w302 w365 w405 w471 _ _ _ w708 w736 w873 w900] -> w102
      tunnel: w101 -> [_ _ _ w243 w302 w365 w405 w471 _ _ _ _ w736 w873 w900]
      tunnel: [w165 w205 w221 w248 w311 w374 w419 w472 w560 w612 w654 w709 w743 w882 w903] -> w100
      tunnel: w93 -> [_ _ _ _ _ _ w423 _ _ _ _ _ w760 _ _]
      tunnel: w72 -> [_ w194 _ _ _ _ w417 _ _ _ _ _ w754 _ _]
      tunnel: w83 -> [_ _ _ _ _ _ w420 _ _ _ _ _ w753 _ _]
      tunnel: w81 -> [_ _ _ _ w304 _ _ _ _ _ _ _ _ _ _]
      tunnel: "Waste Port (Valve 4)" -> [_ _ _ _ _ _ _ _ _ _ _ _ w746 _ _]
      tunnel: [_ _ _ w242 w300 w363 w408 _ _ _ _ w701 w731 w872 w902] -> w77
      tunnel: [_ _ _ w241 w301 w364 w407 _ _ _ _ w700 w730 w871 w901] -> w76
      tunnel: w75 -> [_ _ _ w241 w301 w364 w407 _ _ _ _ _ w730 w871 w901]
      tunnel: w74 -> [_ _ _ w242 w300 w363 w408 _ _ _ _ _ w731 w872 w902]
      frame "Start operation", Default {
        w163 = FALSE ("Pumping")
        n43 = call "initialise Channel.vi"("error in (no error)"=w170, "channel"=u32 0) -> ("error out"=w169:errorcluster)  [unwired: 8 in, 1 out]
        n44 = flat-sequence {
          tunnel: w169 -> [w189]
          tunnel: [w189] -> w166
          frame #0 {
            n45 = Wait (ms)(milliseconds to wait=u32 1000) -> ()  [unwired: 1 out]
          }
        }
        n46 = Greater Than 0?(x=w185) -> (x > 0?=w184:bool)
        n47 = case shown="False" w184 {
          tunnel: [SPS_Flow_System_Automation_Control."Start operation" SPS_Flow_System_Automation_Control."Initialize"] -> w183
          tunnel: [TRUE _] -> w181
          frame False {
            n48 = One Button Dialog(message="No entries found in the table.\n\nPlease add at least 1 entry in the spreadsheet before starting the operation.") -> ()  [unwired: 1 in, 1 out]
          }
          frame True {
          }
        }
        n49 = call "initialise Channel.vi"("error in (no error)"=w166, "channel"=u32 1) -> ("error out"=w164:errorcluster)  [unwired: 8 in, 1 out]
        n50 = flat-sequence {
          tunnel: w164 -> [w187]
          tunnel: [w187] -> w165
          frame #0 {
            n51 = Wait (ms)(milliseconds to wait=u32 1000) -> ()  [unwired: 1 out]
          }
        }
        n52 = local write "Pump2-1"(w163) -> ()
        n53 = local write "Pump2-2"(w163) -> ()
        n54 = local write "Pump1"(w163) -> ()
      }
      frame "Initialize" {
        # "Stay at Initialize state until both channels are initialized"
        n55 = Equal?(x=2, y=w215) -> (x = y?=w197:bool)
        n56 = Equal?(x=2, y=w194) -> (x = y?=w196:bool)
        n57 = And(x=w197, y=w196) -> (x .and. y?=w195:bool)
        n58 = Select(t=SPS_Flow_System_Automation_Control."Wait to start", s=w195, f=SPS_Flow_System_Automation_Control."Initialize") -> (s? t:f=w213:T1)
      }
      frame "Wait to start" {
        w218 = T4."Enabled" ("Disabled")
        n59 = property on="stop" class="Bool"("DisabledEnum"=w218) -> ()  [unwired: 2 in, 2 out]
        n60 = property on="Start" class="Bool (strict)"("DisabledEnum"=w218) -> ()  [unwired: 2 in, 2 out]
        n61 = Select(t=SPS_Flow_System_Automation_Control."Set valves position", s="Start", f=SPS_Flow_System_Automation_Control."Wait to start") -> (s? t:f=w216:T1)
      }
      frame "Set valves position" {
        n62 = To Unsigned Long Integer(number=w284) -> (unsigned 32bit integer=w283:u32)
        n63 = To Unsigned Long Integer(number=w244) -> (unsigned 32bit integer=w282:u32)
        n64 = To Unsigned Long Integer(number=w245) -> (unsigned 32bit integer=w280:u32)
        n65 = To Unsigned Long Integer(number=w246) -> (unsigned 32bit integer=w255:u32)
        n66 = call "Set Actuator Position.vi"("error in (no error)"=w264, "Position (1 to NP)"=w283, "VISA resource name"=w281) -> ("error out"=w239:errorcluster, "VISA resource name out"=w240:refnum<visa-resource-name>)  [unwired: 7 in]
        n67 = call "Set Actuator Position.vi"("error in (no error)"=w258, "Position (1 to NP)"=w255, "VISA resource name"=w259) -> ("error out"=w233:errorcluster, "VISA resource name out"=w234:refnum<visa-resource-name>)  [unwired: 7 in]
        n68 = call "Set Actuator Position.vi"("error in (no error)"=w286, "Position (1 to NP)"=w282, "VISA resource name"=w289) -> ("error out"=w237:errorcluster, "VISA resource name out"=w238:refnum<visa-resource-name>)  [unwired: 7 in]
        n69 = call "Set Actuator Position.vi"("error in (no error)"=w287, "Position (1 to NP)"=w280, "VISA resource name"=w288) -> ("error out"=w235:errorcluster, "VISA resource name out"=w236:refnum<visa-resource-name>)  [unwired: 7 in]
        n70 = call "Get Current Position.vi"("error in (no error)"=w239, "VISA resource name"=w240) -> ("Current Position out"=w285:u32, "VISA resource name out"=w279:refnum<visa-resource-name>)  [unwired: 7 in, 1 out]
        n71 = call "Get Current Position.vi"("error in (no error)"=w237, "VISA resource name"=w238) -> ("Current Position out"=w276:u32, "VISA resource name out"=w272:refnum<visa-resource-name>)  [unwired: 7 in, 1 out]
        n72 = call "Get Current Position.vi"("error in (no error)"=w235, "VISA resource name"=w236) -> ("Current Position out"=w275:u32, "VISA resource name out"=w271:refnum<visa-resource-name>)  [unwired: 7 in, 1 out]
        n73 = call "Get Current Position.vi"("error in (no error)"=w233, "VISA resource name"=w234) -> ("Current Position out"=w256:u32, "VISA resource name out"=w254:refnum<visa-resource-name>)  [unwired: 7 in, 1 out]
        n74 = property on="stop" class="Bool"("DisabledEnum"=T4."Enabled" ("Disabled")) -> ()  [unwired: 2 in, 2 out]
        n75 = Equal?(x=w255, y=w256) -> (x = y?=w257:bool)
        n76 = Equal?(x=w283, y=w285) -> (x = y?=w278:bool)
        n77 = Equal?(x=w282, y=w276) -> (x = y?=w274:bool)
        n78 = Equal?(x=w280, y=w275) -> (x = y?=w273:bool)
        n79 = Bundle(cluster=cluster{i32, i32} {0, 0}, w265, -2) -> (w267:cluster{i32, i32})
        n80 = Compound Arithmetic op=AND(w278, w274, w273, w257) -> (w263:bool)
        n81 = property on="Conditions Table" class="Tbl (strict)"("Active Cell"=w267, "Cell BG Color"=u32 14483200) -> ()  [unwired: 2 in, 2 out]
        n82 = Or(x=w263, y="Valve pos reached") -> (x .or. y?=w261:bool)
        n83 = Select(t=SPS_Flow_System_Automation_Control."Turn on heating", s=w261, f=SPS_Flow_System_Automation_Control."Set valves position") -> (s? t:f=w247:T1)
      }
      frame "Turn on heating" {
        # "If duration = 0 (off): need to wait to reach temp\notherwise: fill syringe/start pumps"
        # "If Q2-1 or Q2-2 is nonzero and valve2 position changes from previous row: need to fill syringe\notherwise: start pumping"
        n84 = To Unsigned Word Integer(number=w303) -> (unsigned 16bit integer=w310:u16)
        n85 = To Unsigned Word Integer(number=w304) -> (unsigned 16bit integer=w305:u16)
        n86 = Equal To 0?(x=w309) -> (x = 0?=w308:bool)
        n87 = Equal To 0?(x=w310) -> (x = 0?=w292:bool)
        n88 = case shown="True" w292 {
          tunnel: w315 -> [w355 w362]
          tunnel: w314 -> [w354 w361]
          tunnel: w310 -> [w353 _]
          tunnel: [w348 w360] -> w296
          tunnel: [w347 w359] -> w295
          frame False {
            n89 = call "Enter set temperature in Celcius.vi"("error in (no error)"=w354, "Temperature (C)"=w353, "VISA resource name"=w355) -> ("error out"=w351:errorcluster, "VISA resource name out"=w350:refnum<visa-resource-name>)  [unwired: 7 in]
            n90 = flat-sequence {
              tunnel: w351 -> [w357]
              tunnel: [w357] -> w352
              tunnel: w350 -> [w356]
              tunnel: [w356] -> w349
              frame #0 {
                n91 = Wait (ms)(milliseconds to wait=u32 100) -> ()  [unwired: 1 out]
              }
            }
            n92 = call "Start heater control.vi"("error in (no error)"=w352, "VISA resource name"=w349) -> ("error out"=w347:errorcluster, "VISA resource name out"=w348:refnum<visa-resource-name>)  [unwired: 8 in]
          }
          frame True {
            n93 = call "Stop heater control.vi"("error in (no error)"=w361, "VISA resource name"=w362) -> ("error out"=w359:errorcluster, "VISA resource name out"=w360:refnum<visa-resource-name>)  [unwired: 8 in]
          }
        }
        n94 = flat-sequence {
          tunnel: w295 -> [w326]
          tunnel: [w326] -> w294
          tunnel: [w325] -> w293
          tunnel: w296 -> [w325]
          frame #0 {
            n95 = Wait (ms)(milliseconds to wait=u32 100) -> ()  [unwired: 1 out]
          }
        }
        n96 = Equal To 0?(x=w305) -> (x = 0?=w291:bool)
        n97 = case shown="False" w291 {
          tunnel: w305 -> [w339 _]
          tunnel: [w334 w344] -> w298
          tunnel: [w333 w343] -> w297
          tunnel: w294 -> [w332 w345]
          tunnel: w293 -> [w331 w346]
          frame False {
            n98 = call "Enter set motor speed in rpm.vi"("error in (no error)"=w332, "Motor speed (10rpm)"=w339, "VISA resource name"=w331) -> ("error out"=w338:errorcluster, "VISA resource name out"=w336:refnum<visa-resource-name>)  [unwired: 7 in]
            n99 = flat-sequence {
              tunnel: w338 -> [w341]
              tunnel: [w341] -> w337
              tunnel: [w340] -> w335
              tunnel: w336 -> [w340]
              frame #0 {
                n100 = Wait (ms)(milliseconds to wait=u32 100) -> ()  [unwired: 1 out]
              }
            }
            n101 = call "Start motor.vi"("error in (no error)"=w337, "VISA resource name"=w335) -> ("error out"=w333:errorcluster, "VISA resource name out"=w334:refnum<visa-resource-name>)  [unwired: 8 in]
          }
          frame True {
            n102 = call "Stop motor.vi"("error in (no error)"=w345, "VISA resource name"=w346) -> ("error out"=w343:errorcluster, "VISA resource name out"=w344:refnum<visa-resource-name>)  [unwired: 8 in]
          }
        }
        n103 = flat-sequence {
          tunnel: w297 -> [w329]
          tunnel: [w329] -> w312
          tunnel: [w328] -> w313
          tunnel: w298 -> [w328]
          frame #0 {
            n104 = Wait (ms)(milliseconds to wait=u32 100) -> ()  [unwired: 1 out]
          }
        }
        n105 = Select(t=SPS_Flow_System_Automation_Control."Wait to reach temp", s=w308, f=SPS_Flow_System_Automation_Control."Fill syringe pump") -> (s? t:f=w306:T1)
      }
      frame "Wait to reach temp" {
        w367 = TRUE ("Auto Reset")
        w373 = 1.0 ("y")
        # "Pause the timer"
        n106 = Add(x=w366, y=w373) -> (x+y=w382:dbl)
        n107 = Subtract(x=w366, y=w373) -> (x-y=w381:dbl)
        n108 = In Range and Coerce(upper limit=w382, x=w378, lower limit=w381) -> (In Range?=w380:bool)  [unwired: 1 out]
        n109 = Or(x=w380, y="temp reached") -> (x .or. y?=w383:bool)
        n110 = call "Elapsed Time (Pause timer)"("Reset"=w367, "Auto Reset"=w367) -> ("Present (s)"=w372:dbl)  [unwired: 10 in, 7 out]
        n111 = Select(t=SPS_Flow_System_Automation_Control."Resume pumps", s=w383, f=SPS_Flow_System_Automation_Control."Wait to reach temp") -> (s? t:f=w392:T1)
        n112 = Subtract(x=w372, y=w371) -> (x-y=w368:dbl)
        n113 = Add(x=w368, y=w370) -> (x+y=w369:dbl)
      }
      frame "Fill syringe pump" {
        # "if Q2_cur !=0:\n    if valve2_cur != valve2_prev: \n        Fill\n    else if Q2_prev = 0:\n            Fill\nelse: Do not fill"
        # "Two cases where the Asia pump needs to fill the syringe before pumping:\n1.  Current flowrate is nonzero, and the valve2 position has changed from the previous row\n2.  Current flowrate is nonzero, and the valve2 position is the same as the previous row, but the previous flowrate is zero, i.e. the pump did not run in previous row and it is not filled with solution."
        n114 = Not Equal To 0?(x=w410) -> (x != 0?=w404:bool)
        n115 = Not Equal To 0?(x=w409) -> (x != 0?=w398:bool)
        n116 = Equal?(x=w406, y=w405) -> (x = y?=w396:bool)
        n117 = Equal To 0?(x=w408) -> (x = 0?=w402:bool)
        n118 = Not(x=w396) -> (.not. x?=w395:bool)
        n119 = And(x=w396, y=w402) -> (x .and. y?=w401:bool)
        n120 = Equal To 0?(x=w407) -> (x = 0?=w397:bool)
        n121 = Or(x=w395, y=w401) -> (x .or. y?=w400:bool)
        n122 = And(x=w404, y=w400) -> (x .and. y?=w403:bool)
        n123 = case shown="True" w403 {
          tunnel: w423 -> [_ w460]
          tunnel: w422 -> [w454 w458]
          tunnel: [w454 w456] -> w421
          tunnel: w418 -> [_ w459]
          tunnel: [TRUE w455] -> w416
          frame False {
            # "If no need to fill"
          }
          frame True {
            # "If need to fill"
            n124 = call "Asia set maximum flowrate (SubVI).vi"("Syringe Diam"=w460) -> ("Max Flowrate"=w457:sgl)  [unwired: 10 in]
            n125 = case shown="4" w459 {
              tunnel: [_ TRUE _] -> w455
              tunnel: w458 -> [w463 w465 w468]
              tunnel: [w462 w465 w469] -> w456
              tunnel: w457 -> [w461 _ w467]
              frame 2, Default {
                # "Idle"
                n126 = call "fill.vi"("error in (no error)"=w463, "rate"=w461, "channel"=u32 0) -> ("error out"=w462:errorcluster)  [unwired: 7 in, 1 out]
              }
              frame 4 {
                # "Full"
              }
              frame 6 {
                # "Empty"
                n127 = call "fill.vi"("error in (no error)"=w468, "rate"=w467, "channel"=u32 0) -> ("error out"=w469:errorcluster)  [unwired: 7 in, 1 out]
              }
            }
          }
        }
        n128 = And(x=w396, y=w397) -> (x .and. y?=w394:bool)
        n129 = Or(x=w395, y=w394) -> (x .or. y?=w393:bool)
        n130 = And(x=w398, y=w393) -> (x .and. y?=w399:bool)
        n131 = case shown="True" w399 {
          tunnel: w421 -> [w436 w440]
          tunnel: w420 -> [_ w442]
          tunnel: [w436 w441] -> w419
          tunnel: w417 -> [_ w438]
          tunnel: [TRUE w437] -> w415
          frame False {
            # "If no need to fill"
          }
          frame True {
            # "If need to fill"
            n132 = call "Asia set maximum flowrate (SubVI).vi"("Syringe Diam"=w442) -> ("Max Flowrate"=w439:sgl)  [unwired: 10 in]
            n133 = case shown="6" w438 {
              tunnel: [_ TRUE _] -> w437
              tunnel: w440 -> [w445 w447 w450]
              tunnel: [w444 w447 w451] -> w441
              tunnel: w439 -> [w443 _ w449]
              frame 2, Default {
                # "Idle"
                n134 = call "fill.vi"("error in (no error)"=w445, "rate"=w443, "channel"=u32 1) -> ("error out"=w444:errorcluster)  [unwired: 7 in, 1 out]
              }
              frame 4 {
                # "Full"
              }
              frame 6 {
                # "Empty"
                n135 = call "fill.vi"("error in (no error)"=w450, "rate"=w449, "channel"=u32 1) -> ("error out"=w451:errorcluster)  [unwired: 7 in, 1 out]
              }
            }
          }
        }
        n136 = And(x=w416, y=w415) -> (x .and. y?=w414:bool)
        n137 = Select(t=SPS_Flow_System_Automation_Control."Start pumps", s=w414, f=SPS_Flow_System_Automation_Control."Fill syringe pump") -> (s? t:f=w411:T1)
      }
      frame "Start pumps" {
        # "Start the timer"
        n138 = Equal To 0?(x=w478) -> (x = 0?=w480:bool)
        n139 = To Single Precision Float(number=w478) -> (single precision float=w479:sgl)
        n140 = case shown="False" w480 {
          tunnel: w477 -> [w512 w515]
          tunnel: w479 -> [w510 _]
          tunnel: [w508 w514] -> w473
          frame False {
            # "If flowrate2-left is nonzero, start pumping"
            n141 = call "pump.vi"("error in (no error)"=w512, "rate"=w510, "channel"=u32 0) -> ("error out"=w508:errorcluster)  [unwired: 7 in, 1 out]
            n142 = Wait (ms)(milliseconds to wait=u32 100) -> ()  [unwired: 1 out]
            "Pump2-1" <- TRUE ("Pump2-1")
          }
          frame True {
            # "If flowrate2-left is zero, stop pumping"
            n143 = call "pump Stop.vi"("error in (no error)"=w515, "channel"=u32 0) -> ("error out"=w514:errorcluster)  [unwired: 8 in, 1 out]
            n144 = local write "Pump2-1"(FALSE) -> ()
            n145 = Wait (ms)(milliseconds to wait=u32 100) -> ()  [unwired: 1 out]
          }
        }
        n146 = Equal To 0?(x=w474) -> (x = 0?=w476:bool)
        n147 = To Single Precision Float(number=w474) -> (single precision float=w475:sgl)
        n148 = Equal To 0?(x=w485) -> (x = 0?=w482:bool)
        n149 = case shown="True" w476 {
          tunnel: w473 -> [w501 w505]
          tunnel: w475 -> [w499 _]
          tunnel: [w497 w502] -> w472
          frame False {
            # "If flowrate2-left is nonzero, start pumping"
            n150 = call "pump.vi"("error in (no error)"=w501, "rate"=w499, "channel"=u32 1) -> ("error out"=w497:errorcluster)  [unwired: 7 in, 1 out]
            n151 = Wait (ms)(milliseconds to wait=u32 100) -> ()  [unwired: 1 out]
            "Pump2-2" <- TRUE ("Pump2-1")
          }
          frame True {
            # "If flowrate2-left is zero, stop pumping"
            n152 = call "pump Stop.vi"("error in (no error)"=w505, "channel"=u32 1) -> ("error out"=w502:errorcluster)  [unwired: 8 in, 1 out]
            n153 = local write "Pump2-2"(FALSE) -> ()
            n154 = Wait (ms)(milliseconds to wait=u32 100) -> ()  [unwired: 1 out]
          }
        }
        n155 = case shown="False" w482 {
          tunnel: w494 -> [w523 w538]
          tunnel: w493 -> [w522 w535]
          tunnel: w485 -> [w521 _]
          tunnel: [w520 w537] -> w484
          tunnel: [w519 w536] -> w483
          frame False {
            # "If flowrate1 is nonzero, start pumping"
            n156 = disable-structure shown="Enabled" {
              disable-tunnel: w523 -> [w530 _]
              disable-tunnel: w522 -> [w529 _]
              disable-tunnel: w521 -> [w528 _]
              disable-tunnel: [w527 _] -> w520
              disable-tunnel: [w526 _] -> w519
              frame Enabled {
                n157 = call "Configure Flowrate.vi"("error in (no error)"=w529, "Flowrate (1 ml/min)"=w528, "VISA resource name"=w530) -> ("error out"=w525:errorcluster, "VISA resource name out"=w531:refnum<visa-resource-name>)  [unwired: 7 in]
                n158 = flat-sequence {
                  tunnel: w525 -> [w532]
                  tunnel: [w532] -> w524
                  frame #0 {
                    n159 = Wait (ms)(milliseconds to wait=u32 100) -> ()  [unwired: 1 out]
                  }
                }
                n160 = call "Start.vi"("error in (no error)"=w524, "VISA resource name"=w531) -> ("error out"=w526:errorcluster, "VISA resource name out"=w527:refnum<visa-resource-name>)  [unwired: 8 in]
              }
              frame Disabled {
              }
            }
            "Pump1" <- TRUE
          }
          frame True {
            # "If flowrate1 is zero, stop pumping"
            n161 = disable-structure shown="Enabled" {
              disable-tunnel: w538 -> [w542 _]
              disable-tunnel: [w541 _] -> w537
              disable-tunnel: [w540 _] -> w536
              disable-tunnel: w535 -> [w539 _]
              frame Enabled {
                n162 = call "Stop.vi"("error in (no error)"=w539, "VISA resource name"=w542) -> ("error out"=w540:errorcluster, "VISA resource name out"=w541:refnum<visa-resource-name>)  [unwired: 8 in]
              }
              frame Disabled {
              }
            }
            n163 = local write "Pump1"(FALSE) -> ()
          }
        }
        n164 = call "Elapsed Time (Start)"() -> ("Present (s)"=w489:dbl)  [unwired: 12 in, 7 out]
      }
      frame "Check temp & time " {
        w574 = TRUE
        # "If pause button is on OR (set temp != 0 but temp is out of range: Need to pause"
        # "Pause clock"
        n165 = local read "temp reached"() -> (w545:bool)
        n166 = Add(x=w557, y="Temp range") -> (x+y=w573:dbl)
        n167 = Subtract(x=w557, y="Temp range") -> (x-y=w572:dbl)
        n168 = Not Equal To 0?(x=w557) -> (x != 0?=w549:bool)
        n169 = In Range and Coerce(upper limit=w573, x=w562, lower limit=w572) -> (In Range?=w546:bool)  [unwired: 1 out]
        n170 = Multiply(x=w585, y=60.0) -> (x*y=w584:dbl)
        n171 = Or(x=w546, y=w545) -> (x .or. y?=w547:bool)
        n172 = Not(x=w547) -> (.not. x?=w550:bool)
        n173 = property on="Pause" class="Bool (strict)"("DisabledEnum"=T4."Enabled" ("Disabled")) -> ()  [unwired: 2 in, 2 out]
        n174 = call "Elapsed Time"("Time Target (s)"=w584, "Reset"=w574, "Auto Reset"=w574, "Set Start Time (s)"=w563) -> ("Present (s)"=w575:dbl, "Elapsed Time (s)"=w556:dbl, "Time has Elapsed"=w578:bool)  [unwired: 8 in, 5 out]
        n175 = And(x=w549, y=w550) -> (x .and. y?=w548:bool)
        n176 = Less?(x=w556, y=1.0) -> (x < y?=w553:bool)
        n177 = Divide(x=w556, y=60.0) -> (x/y=w544:dbl)
        n178 = Select(t=0.0 ("f"), s=w553, f=w544) -> (s? t:f=→"Elapsed Time":dbl)
        n179 = Or(x=w548, y="Pause") -> (x .or. y?=w570:bool)
        n180 = Select(t=SPS_Flow_System_Automation_Control."Stop pumps", s=w578, f=SPS_Flow_System_Automation_Control."Check temp & time ") -> (s? t:f=w569:T1)
        n181 = case shown="False" w570 {
          tunnel: [w590 w595] -> w577
          tunnel: [w592 w596] -> w576
          tunnel: w575 -> [w590 w595]
          tunnel: w578 -> [w591 _]
          tunnel: w563 -> [w589 w593]
          tunnel: w561 -> [_ w594]
          frame False {
            n182 = Select(t=w590, s=w591, f=w589) -> (s? t:f=w592:dbl)
          }
          frame True {
            n183 = Subtract(x=w595, y=w594) -> (x-y=w597:dbl)
            n184 = Add(x=w597, y=w593) -> (x+y=w596:dbl)
          }
        }
        n185 = Select(t=SPS_Flow_System_Automation_Control."Pause pumps ", s=w570, f=w569) -> (s? t:f=w567:T1)
      }
      frame "Pause pumps " {
        w606 = TRUE ("Auto Reset")
        # "If the user paused the program by pressing pause button: stay in current state\nif the program is pause because temperature is out of range: go to wait to reach temp"
        # "Pause the timer"
        n186 = local read "Pump1"() -> (w601:bool)
        n187 = local read "Pump2-1"() -> (w600:bool)
        n188 = local read "Pump2-2"() -> (w599:bool)
        n189 = Compound Arithmetic op=OR(w601, w600, w599) -> (w598:bool)
        n190 = case shown="True" w598 {
          tunnel: w624 -> [w627 w634]
          tunnel: w623 -> [w626 w633]
          tunnel: [w627 w632] -> w621
          tunnel: [w626 w631] -> w618
          tunnel: w613 -> [w625 w630]
          tunnel: [w625 w629] -> w612
          frame False {
            # "else: nothing"
          }
          frame True {
            w628 = FALSE ("Pump")
            # "If any pump is pumping, stop them"
            n191 = disable-structure shown="Enabled" {
              disable-tunnel: w634 -> [w644 _]
              disable-tunnel: w633 -> [w643 _]
              disable-tunnel: [w642 _] -> w632
              disable-tunnel: [w641 _] -> w631
              disable-tunnel: w630 -> [w640 _]
              disable-tunnel: [w638 _] -> w629
              frame Enabled {
                n192 = call "pump Stop.vi"("error in (no error)"=w640, "channel"=u32 0) -> ("error out"=w636:errorcluster)  [unwired: 8 in, 1 out]
                n193 = call "Stop.vi"("error in (no error)"=w643, "VISA resource name"=w644) -> ("error out"=w641:errorcluster, "VISA resource name out"=w642:refnum<visa-resource-name>)  [unwired: 8 in]
                n194 = flat-sequence {
                  tunnel: w636 -> [w646]
                  tunnel: [w646] -> w635
                  frame #0 {
                    n195 = Wait (ms)(milliseconds to wait=u32 100) -> ()  [unwired: 1 out]
                  }
                }
                n196 = call "pump Stop.vi"("error in (no error)"=w635, "channel"=u32 1) -> ("error out"=w638:errorcluster)  [unwired: 8 in, 1 out]
              }
              frame Disabled {
              }
            }
            n197 = local write "Pump1"(w628) -> ()
            n198 = local write "Pump2-1"(w628) -> ()
            n199 = local write "Pump2-2"(w628) -> ()
          }
        }
        n200 = local read "Pause"() -> (w608:bool)
        n201 = Select(t=SPS_Flow_System_Automation_Control."Pause pumps ", s=w608, f=SPS_Flow_System_Automation_Control."Wait to reach temp") -> (s? t:f=w611:T1)
        n202 = call "Elapsed Time (Pause timer)2"("Reset"=w606, "Auto Reset"=w606) -> ("Present (s)"=w604:dbl)  [unwired: 10 in, 7 out]
        n203 = Subtract(x=w604, y=w605) -> (x-y=w607:dbl)
        n204 = Add(x=w607, y=w603) -> (x+y=w602:dbl)
      }
      frame "Resume pumps" {
        n205 = To Single Precision Float(number=w656) -> (single precision float=w652:sgl)
        n206 = Not Equal To 0?(x=w656) -> (x != 0?=w649:bool)
        n207 = local write "Pump2-1"(w649) -> ()
        n208 = case shown="True" w649 {
          tunnel: w653 -> [w695 w699]
          tunnel: w652 -> [_ w698]
          tunnel: [w694 w696] -> w651
          frame False {
            n209 = call "pump Stop.vi"("error in (no error)"=w695, "channel"=u32 0) -> ("error out"=w694:errorcluster)  [unwired: 8 in, 1 out]
          }
          frame True {
            n210 = call "pump.vi"("error in (no error)"=w699, "rate"=w698, "channel"=u32 0) -> ("error out"=w696:errorcluster)  [unwired: 7 in, 1 out]
          }
        }
        n211 = Not Equal To 0?(x=w655) -> (x != 0?=w648:bool)
        n212 = To Single Precision Float(number=w655) -> (single precision float=w650:sgl)
        n213 = Not Equal To 0?(x=w662) -> (x != 0?=w647:bool)
        n214 = case shown="False" w648 {
          tunnel: w651 -> [w688 w692]
          tunnel: w650 -> [_ w691]
          tunnel: [w686 w689] -> w654
          frame False {
            n215 = call "pump Stop.vi"("error in (no error)"=w688, "channel"=u32 1) -> ("error out"=w686:errorcluster)  [unwired: 8 in, 1 out]
          }
          frame True {
            n216 = call "pump.vi"("error in (no error)"=w692, "rate"=w691, "channel"=u32 1) -> ("error out"=w689:errorcluster)  [unwired: 7 in, 1 out]
          }
        }
        n217 = local write "Pump2-2"(w648) -> ()
        n218 = local write "Pump1"(w647) -> ()
        n219 = case shown="True" w647 {
          tunnel: w666 -> [w675 w682]
          tunnel: w665 -> [w672 w681]
          tunnel: w662 -> [_ w680]
          tunnel: [w674 w679] -> w663
          tunnel: [w673 w678] -> w664
          frame False {
            n220 = call "Stop.vi"("error in (no error)"=w672, "VISA resource name"=w675) -> ("error out"=w673:errorcluster, "VISA resource name out"=w674:refnum<visa-resource-name>)  [unwired: 8 in]
          }
          frame True {
            n221 = call "Configure Flowrate.vi"("error in (no error)"=w681, "Flowrate (1 ml/min)"=w680, "VISA resource name"=w682) -> ("error out"=w677:errorcluster, "VISA resource name out"=w683:refnum<visa-resource-name>)  [unwired: 7 in]
            n222 = flat-sequence {
              tunnel: w677 -> [w684]
              tunnel: [w684] -> w676
              frame #0 {
                n223 = Wait (ms)(milliseconds to wait=u32 100) -> ()  [unwired: 1 out]
              }
            }
            n224 = call "Start.vi"("error in (no error)"=w676, "VISA resource name"=w683) -> ("error out"=w678:errorcluster, "VISA resource name out"=w679:refnum<visa-resource-name>)  [unwired: 8 in]
          }
        }
      }
      frame "Stop pumps" {
        w707 = FALSE ("Pumping")
        n225 = call "pump Stop.vi"("error in (no error)"=w710, "channel"=u32 0) -> ("error out"=w706:errorcluster)  [unwired: 8 in, 1 out]
        n226 = flat-sequence {
          tunnel: w706 -> [w729]
          tunnel: [w729] -> w705
          frame #0 {
            n227 = Wait (ms)(milliseconds to wait=u32 100) -> ()  [unwired: 1 out]
          }
        }
        n228 = call "Stop.vi"("error in (no error)"=w717, "VISA resource name"=w719) -> ("error out"=w716:errorcluster, "VISA resource name out"=w718:refnum<visa-resource-name>)  [unwired: 8 in]
        n229 = call "pump Stop.vi"("error in (no error)"=w705, "channel"=u32 1) -> ("error out"=w709:errorcluster)  [unwired: 8 in, 1 out]
        n230 = Bundle(w722, -2) -> (w724:cluster{i32, i32})  [unwired: 1 in]
        n231 = property on="Conditions Table" class="Tbl (strict)"("Active Cell"=w724, "Cell BG Color"=u32 13816530) -> ()  [unwired: 2 in, 2 out]
        n232 = Increment(x=w722) -> (x+1=w720:i32)
        n233 = local write "Pump1"(w707) -> ()
        n234 = local write "Pump2-1"(w707) -> ()
        n235 = local write "Pump2-2"(w707) -> ()
      }
      frame "Empty syringe pump" {
        # "Two cases where the Asia pump needs to empty the syringe before going to next row: \n1. Current flowrate is nonzero but the next flowrate is zero;\n2. Current flowrate is nonzero but valve2 will change position in next row."
        # "If (flowrate != 0) AND (flowrate_next = 0 OR valve2_next != valve2):\n    need to empty\nelse: ready for next state"
        # "If (Left no need to empty OR already emtpy) AND (Right no need to empty OR already empty):\n    go to next state 'Check next step'\nelse: stay in current state 'Empty syringe pump'"
        n236 = Equal To 0?(x=w741) -> (x = 0?=w740:bool)
        n237 = Equal To 0?(x=w742) -> (x = 0?=w739:bool)
        n238 = Not Equal?(x=w763, y=w736) -> (x != y?=w757:bool)
        n239 = Not Equal To 0?(x=w731) -> (x != 0?=w735:bool)
        n240 = Not Equal To 0?(x=w730) -> (x != 0?=w733:bool)
        n241 = Or(x=w740, y=w757) -> (x .or. y?=w734:bool)
        n242 = And(x=w734, y=w735) -> (x .and. y?=w738:bool)
        n243 = Or(x=w739, y=w757) -> (x .or. y?=w732:bool)
        n244 = case shown="False" w738 {
          tunnel: w762 -> [w823 w838]
          tunnel: w761 -> [w822 w837]
          tunnel: [w823 w833] -> w759
          tunnel: w756 -> [_ w832]
          tunnel: w760 -> [_ w826]
          tunnel: [TRUE w831] -> w750
          tunnel: [w822 w830] -> w758
          tunnel: w746 -> [_ w829]
          tunnel: w745 -> [w821 w828]
          tunnel: [w821 w827] -> w744
          frame False {
            # "Left channel no need to empty"
          }
          frame True {
            # "Left channel needs to empty"
            n245 = disable-structure shown="Enabled" {
              disable-tunnel: w838 -> [w844 _]
              disable-tunnel: w837 -> [w843 _]
              disable-tunnel: [w842 TRUE] -> w836
              disable-tunnel: [w841 _] -> w835
              disable-tunnel: [w840 _] -> w834
              disable-tunnel: w829 -> [w839 _]
              frame Enabled {
                n246 = call "Get Current Position.vi"("error in (no error)"=w843, "VISA resource name"=w844) -> ("error out"=w840:errorcluster, "Current Position out"=w845:u32, "VISA resource name out"=w841:refnum<visa-resource-name>)  [unwired: 7 in]
                n247 = Equal?(x=w845, y=w839) -> (x = y?=w842:bool)
              }
              frame Disabled {
              }
            }
            n248 = call "Asia set maximum flowrate (SubVI).vi"("Syringe Diam"=w826) -> ("Max Flowrate"=w825:sgl)  [unwired: 10 in]
            n249 = case shown="True" w836 {
              tunnel: w835 -> [w852 w859]
              tunnel: w834 -> [w851 w855]
              tunnel: w829 -> [w850 _]
              tunnel: [w849 w859] -> w833
              tunnel: w825 -> [_ w858]
              tunnel: w832 -> [_ w857]
              tunnel: [_ w856] -> w831
              tunnel: [w848 w855] -> w830
              tunnel: w828 -> [w847 w854]
              tunnel: [w847 w853] -> w827
              frame False {
                # "Valve4 move to waste port"
                n250 = call "Set Actuator Position.vi"("error in (no error)"=w851, "Position (1 to NP)"=w850, "VISA resource name"=w852) -> ("error out"=w848:errorcluster, "VISA resource name out"=w849:refnum<visa-resource-name>)  [unwired: 7 in]
              }
              frame True {
                # "Valve4 at waste port"
                n251 = case shown="2, Default" w857 {
                  tunnel: w858 -> [w863 w867 _ _]
                  tunnel: [_ _ _ TRUE] -> w856
                  tunnel: w854 -> [w861 w865 w868 w869]
                  tunnel: [w860 w864 w868 w869] -> w853
                  frame 2, Default {
                    # "Idle"
                    n252 = call "empty.vi"("error in (no error)"=w861, "rate"=w863, "channel"=u32 0) -> ("error out"=w860:errorcluster)  [unwired: 7 in, 1 out]
                  }
                  frame 4 {
                    # "Full"
                    n253 = call "empty.vi"("error in (no error)"=w865, "rate"=w867, "channel"=u32 0) -> ("error out"=w864:errorcluster)  [unwired: 7 in, 1 out]
                  }
                  frame 5 {
                    # "Wait for emptying"
                  }
                  frame 6 {
                    # "Empty"
                  }
                }
              }
            }
          }
        }
        n254 = And(x=w732, y=w733) -> (x .and. y?=w737:bool)
        n255 = case shown="True" w737 {
          tunnel: w759 -> [w777 w790]
          tunnel: w758 -> [_ w789]
          tunnel: [w777 w785] -> w755
          tunnel: w754 -> [_ w784]
          tunnel: w753 -> [_ w779]
          tunnel: [TRUE w783] -> w751
          tunnel: w746 -> [_ w782]
          tunnel: w744 -> [w775 w781]
          tunnel: [w775 w780] -> w743
          frame False {
            # "Right channel no need to empty"
          }
          frame True {
            # "Right channel needs to empty"
            n256 = disable-structure shown="Enabled" {
              disable-tunnel: w790 -> [w796 _]
              disable-tunnel: w789 -> [w795 _]
              disable-tunnel: [w794 TRUE] -> w788
              disable-tunnel: [w793 _] -> w787
              disable-tunnel: [w792 _] -> w786
              disable-tunnel: w782 -> [w791 _]
              frame Enabled {
                n257 = call "Get Current Position.vi"("error in (no error)"=w795, "VISA resource name"=w796) -> ("error out"=w792:errorcluster, "Current Position out"=w797:u32, "VISA resource name out"=w793:refnum<visa-resource-name>)  [unwired: 7 in]
                n258 = Equal?(x=w797, y=w791) -> (x = y?=w794:bool)
              }
              frame Disabled {
              }
            }
            n259 = call "Asia set maximum flowrate (SubVI).vi"("Syringe Diam"=w779) -> ("Max Flowrate"=w778:sgl)  [unwired: 10 in]
            n260 = case shown="True" w788 {
              tunnel: w787 -> [w803 w809]
              tunnel: w786 -> [w802 _]
              tunnel: w782 -> [w801 _]
              tunnel: [w800 w809] -> w785
              tunnel: w778 -> [_ w808]
              tunnel: w784 -> [_ w807]
              tunnel: [_ w806] -> w783
              tunnel: w781 -> [w799 w805]
              tunnel: [w799 w804] -> w780
              frame False {
                # "Valve4 move to waste port"
                n261 = call "Set Actuator Position.vi"("error in (no error)"=w802, "Position (1 to NP)"=w801, "VISA resource name"=w803) -> ("VISA resource name out"=w800:refnum<visa-resource-name>)  [unwired: 7 in, 1 out]
              }
              frame True {
                # "Valve4 at waste port"
                n262 = case shown="5" w807 {
                  tunnel: w808 -> [w813 w817 _ _]
                  tunnel: [_ _ _ TRUE] -> w806
                  tunnel: w805 -> [w811 w815 w818 w819]
                  tunnel: [w810 w814 w818 w819] -> w804
                  frame 2, Default {
                    # "Idle"
                    n263 = call "empty.vi"("error in (no error)"=w811, "rate"=w813, "channel"=u32 1) -> ("error out"=w810:errorcluster)  [unwired: 7 in, 1 out]
                  }
                  frame 4 {
                    # "Full"
                    n264 = call "empty.vi"("error in (no error)"=w815, "rate"=w817, "channel"=u32 1) -> ("error out"=w814:errorcluster)  [unwired: 7 in, 1 out]
                  }
                  frame 5 {
                    # "Wait for emptying"
                  }
                  frame 6 {
                    # "Empty"
                  }
                }
              }
            }
          }
        }
        n265 = And(x=w750, y=w751) -> (x .and. y?=w752:bool)
        n266 = property on="Pause" class="Bool (strict)"("DisabledEnum"=T4."Disabled and Grayed Out" ("Disabled")) -> ()  [unwired: 2 in, 2 out]
        n267 = Select(t=SPS_Flow_System_Automation_Control."Check next step", s=w752, f=SPS_Flow_System_Automation_Control."Empty syringe pump") -> (s? t:f=w747:T1)
      }
      frame "Check next step" {
        n268 = Equal To 0?(x=w897) -> (x = 0?=w899:bool)
        n269 = Equal To 0?(x=w896) -> (x = 0?=w898:bool)
        n270 = Equal To 0?(x=w895) -> (x = 0?=w894:bool)
        n271 = Equal To 0?(x=w876) -> (x = 0?=w875:bool)
        n272 = Equal To 0?(x=w877) -> (x = 0?=w874:bool)
        n273 = Compound Arithmetic op=AND(w899, w898, w894, w875, w874) -> (w893:bool)
        n274 = Select(t=SPS_Flow_System_Automation_Control."No more entries", s=w893, f=SPS_Flow_System_Automation_Control."Set valves position") -> (s? t:f=w890:T1)
      }
      frame "No more entries" {
        n275 = One Button Dialog(message="No more entries left. The operation will now stop.") -> ()  [unwired: 1 in, 1 out]
      }
    }
    "State" <- w67
    n276 = Unbundle By Name(w126) -> ("status"=w122:bool)
    n277 = Compound Arithmetic op=OR(w122, w154, "stop", w99, w85) -> (w127:bool)
    n278 = Wait (ms)(milliseconds to wait=u32 10) -> ()  [unwired: 1 out]
  }
  n279 = call "Close.vi"("error in (no error)"=w2, "VISA resource name"=w1) -> ("error out"=w3:errorcluster)  [unwired: 9 in]
  n280 = call "Stop.vi"("error in (no error)"=w39, "VISA resource name"=w40) -> ("error out"=w35:errorcluster)  [unwired: 8 in, 1 out]
  n281 = Not(x=w38) -> (.not. x?=w16:bool)
  n282 = local write "Start"(w16) -> ()
  n283 = local write "Pause"(w16) -> ()
  n284 = local write "Pump1"(w16) -> ()
  n285 = local write "Pump2-1"(w16) -> ()
  n286 = local write "Pump2-2"(w16) -> ()
  n287 = Merge Errors(w35, w3) -> (w34:errorcluster)
  n288 = call "clear Up.vi"("error in (no error)"=w19) -> ("error out"=w18:errorcluster)  [unwired: 10 in]
  n289 = call <vilib>:"Simple Error Handler.vi"("error in (no error)"=w34) -> ()  [unwired: 4 in, 5 out]
  n290 = call "exit Remote Mode.vi"("error in (no error)"=w18) -> ()  [unwired: 9 in, 2 out]
